vi "MicosCore.vi"(5 "NumOfAxis":i32=3, 6 "MotorDisabled":refnum<vi>, 7 "Simulation":bool, 8 "error in":errorcluster, 9 "Serial Configuration":T1={"Baud Rate"=115200, "Parity"=0, "Data Bits"=8, "Stop Bits"=10, "Flow Control"=0} {"Flow Control" items=["None", "XON/XOFF", "RTS/CTS", "XON/XOFF & RTS/CTS", "DTR/DSR", "XON/XOFF & DTR/DSR"]; "Stop Bits" items=["1.0"=10, "1.5"=15, "2.0"=20]; "Data Bits" items=["7"=7, "8"=8]; "Parity" items=["None", "Odd", "Even", "Mark", "Space"]; "Baud Rate" items=["300"=300, "600"=600, "1200"=1200, "2400"=2400, "4800"=4800, "9600"=9600, "19200"=19200]}, 10 "CommPort":refnum<visa-resource-name>, 11 "ControlQueue in":refnum<queue>) -> (0 "error out":errorcluster, 3 "queue out":refnum<queue>)   [LabVIEW 2012, in "Micos_uic.lvlib"]
uses:
  Micos_uic.lvlib
  Public/Data/Micos_State.ctl
  Public/Data/Micos_Data.ctl
  <vilib>/Utility/error.llb/DialogType.ctl
  Public/Position_Micos.vi
  user.lib/Utility/ErrorLog_lib.lvlib
panel:
  out "Numeric":i32
  out "appended array":u32[](array[numeric])
  in  "Go_MoveRel":bool caption="Go"
  out "WaitStopBlink":i32
  out "tick_start":u32
  out "tick_stop":u32
  out "Returned_String":string
  out "refresh rate":i32
  out "resfresh counter":i32
  in  "MotorDisabled":bool caption="Go"
  in  "Home":bool caption="Go"
  in  "StepWidth":dbl(ring)=0.2 items=["0.2 um"=0.0002, "0.001 mm"=0.001, "0.002 mm"=0.002, "0.005 mm "=0.005, "0.01 mm"=0.01, "0.02 mm"=0.02, "0.05 mm"=0.05, "0.1 mm"=0.1, "0.2 mm"=0.2, "1 mm"=1.0]
  in  "Z-":bool
  in  "Z+":bool
  in  "X+":bool
  in  "X-":bool
  in  "Y-":bool
  in  "Y+":bool
  in  "ClearErr":bool caption="Go"
  in  "STOP":bool caption="Go"
  in  "Quit":bool caption="Go"
  out "Instrument Driver Revision":string
  out "Instrument Firmware Revision":string
  in  "SetPosition":dbl[](array[numeric])=[1.0, 1.0, 1.0] caption="Position" format="%.4f"
  in  "SetVelocity":dbl[](array[numeric])=[1.0] caption="Velocity"
  in  "SetAcceleration":dbl[](array[numeric])=[50.0] caption="Acceleration"
  in  "Go":bool
  out "Moving":bool
  out "Acceleration":dbl[](array[numeric])
  out "Velocity":dbl[](array[numeric])
  out "Position":dbl[](array[numeric])
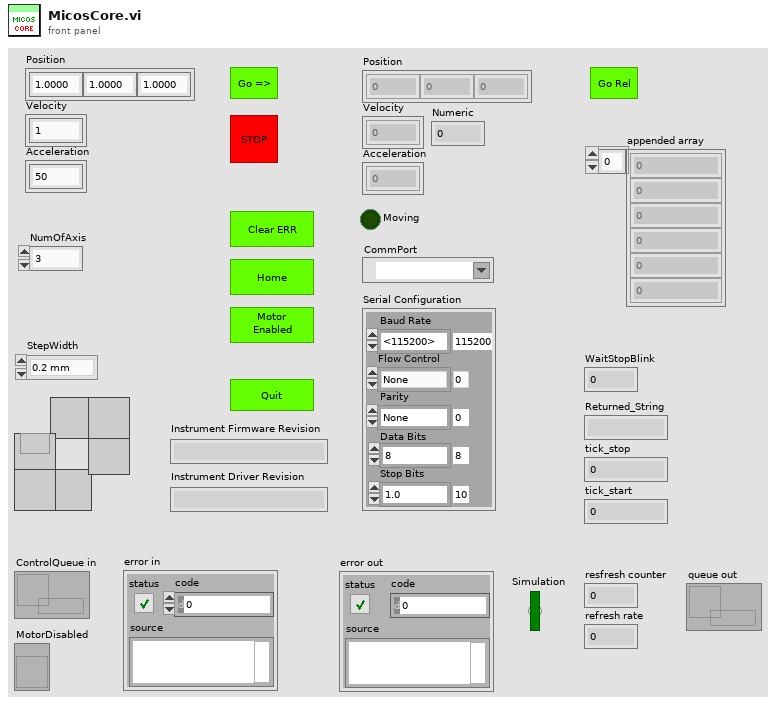
[diagram p1: front panel]
types:
  T1 = cluster{"Baud Rate":u32, "Parity":u16, "Data Bits":u16, "Stop Bits":u16, "Flow Control":u16}
  T2 = cluster{"CommPort":refnum<vi>, "Serial Configuration":refnum<vi>, "SetPosition":refnum<vi>, "SetAcceleration":refnum<vi>, "SetVelocity":refnum<vi>, "StepWidth":refnum<vi>, "WaitStopReturn_Queue":refnum<queue>}
  T3 = typedef "Micos_uic.lvlib/Micos_State.ctl" = cluster{"State":enum16{"Initialize", "SetDefaultConfig", "Close", "Quit", "Identify", "MoveAbs", "MoveAbs_all", "MoveRel", "MoveRel_all", "STOP", "Origin/Home", "WaitStop", "QueryStatus", "UpdateXPos", "UpdateAll", "SetVelocity", "SetAcceleration", "ClearErr", "LogMessage", "MotorEnable(1)", "EnableAxis", "JoyStick", "GetVelocity", "GetAcceleration", "SendCmd", "SetSoftLimits", "Beep", "_SettingReturn"}, "Params.":variant}
  T4 = typedef "Micos_uic.lvlib/Micos_Data.ctl" = cluster{"Position":dbl[], "Velocity":dbl[], "Acceleration":dbl[], "Moving":bool, "Simulation":bool, "tickcount_mov":u32, "tickcount_pos":u32, "NumOfAxis":i32, "Initialized":bool, "CommPort":refnum<visa-resource-name>, "Range":dbl[][], "Serial Configuration":cluster{"Baud Rate":u32, "Parity":u16, "Data Bits":u16, "Stop Bits":u16, "Flow Control":u16}, "MotorDisabled":refnum<vi>}
  T5 = enum16{"Initialize", "SetDefaultConfig", "Close", "Quit", "Identify", "MoveAbs", "MoveAbs_all", "MoveRel", "MoveRel_all", "STOP", "Origin/Home", "WaitStop", "QueryStatus", "UpdateXPos", "UpdateAll", "SetVelocity", "SetAcceleration", "ClearErr", "LogMessage", "MotorEnable(1)", "EnableAxis", "JoyStick", "GetVelocity", "GetAcceleration", "SendCmd", "SetSoftLimits", "Beep", "_SettingReturn"}
  T6 = cluster{"Acceleration":dbl[], "Velocity":dbl[], "tick_move_target":u32, "Position target":dbl[], "Velocity_axial":dbl[]}
  T7 = cluster{"Position_Target":dbl[], "Velocity_axial":dbl[], "Acceleration":dbl[], "Moving":bool, "Simulation":bool, "tick_MoveTarget":u32, "NumOfAxis":i32, "Range":dbl[][]}
  T8 = enum16{"Initialize", "SetDefaultConfig", "Close", "Quit", "Identify", "MoveAbs", "MoveAbs_all", "MoveRel", "MoveRel_all", "STOP", "Origin/Home", "WaitStop", "QueryStatus", "UpdateXPos", "UpdateAll", "SetVelocity", "SetAcceleration", "ClearErr", "LogMessage", "MotorEnable(1)", "EnableAxis", "JoyStick", "GetVelocity", "GetAcceleration", "SendCmd", "SetSoftLimits", "Beep", "_SettingReturn"}[]
  T9 = typedef "DialogType.ctl" = u16
  T10 = typedef "StepWidthSelector.ctl" = dbl
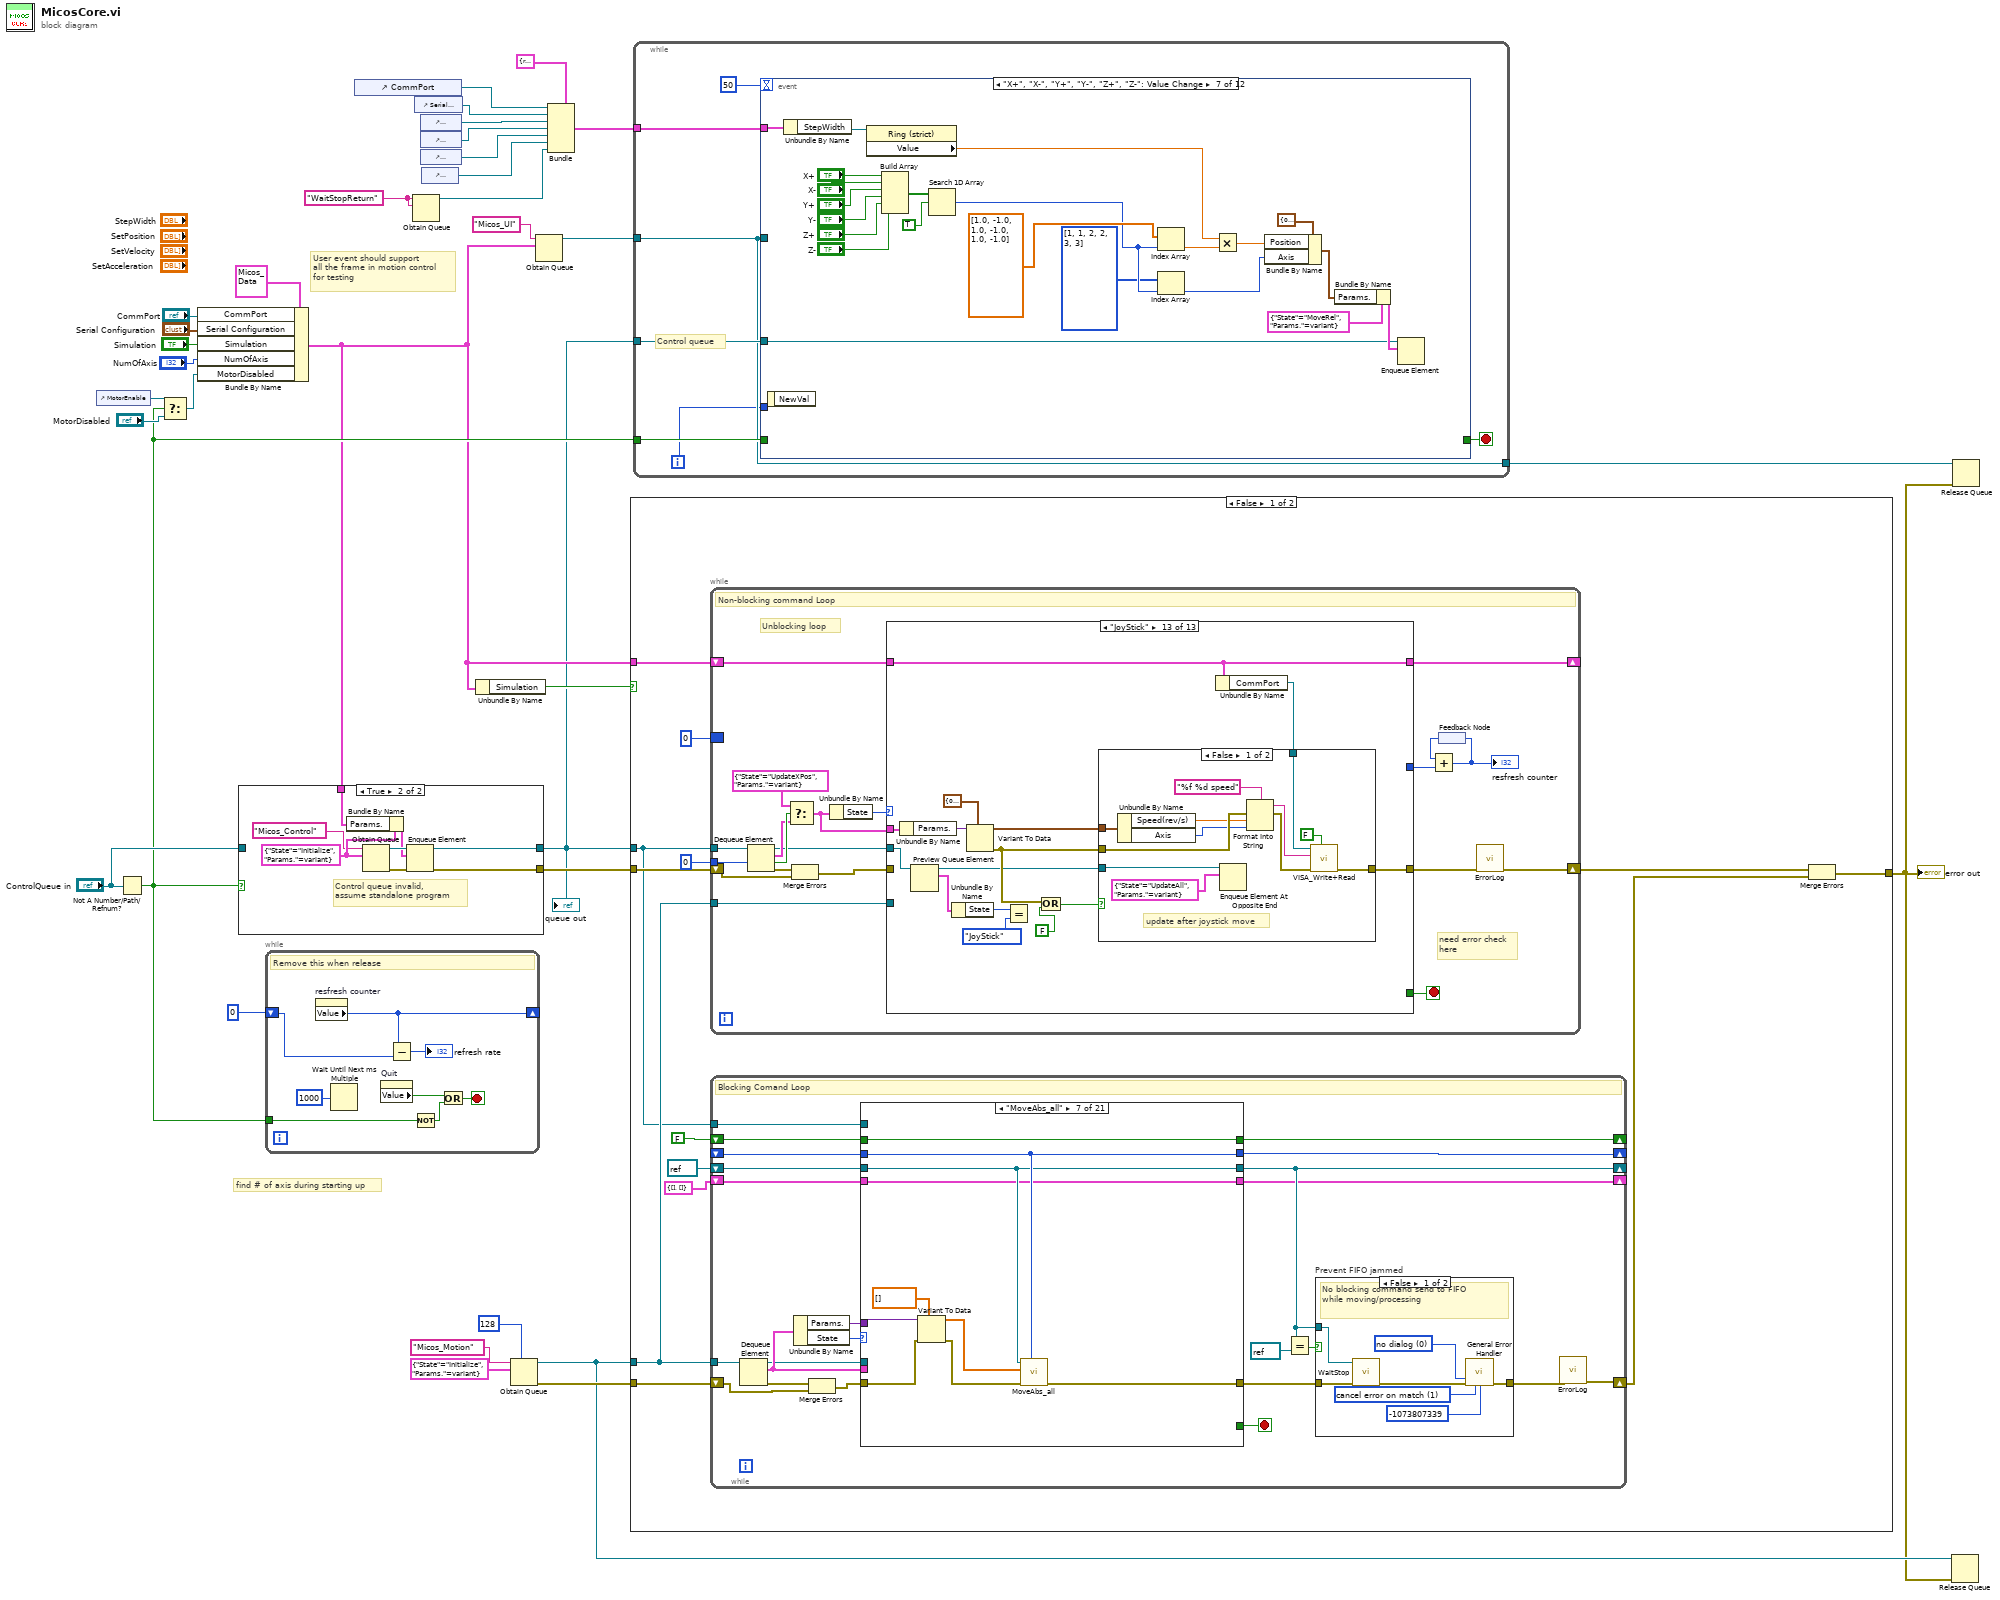
[diagram p0: block diagram]
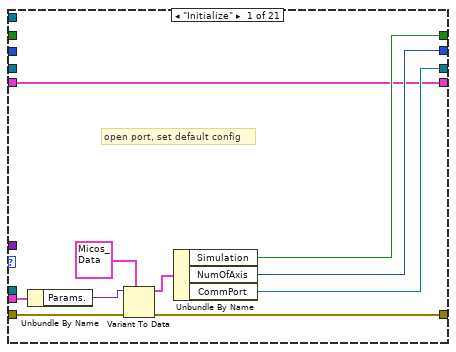
[diagram p3: hidden frame]
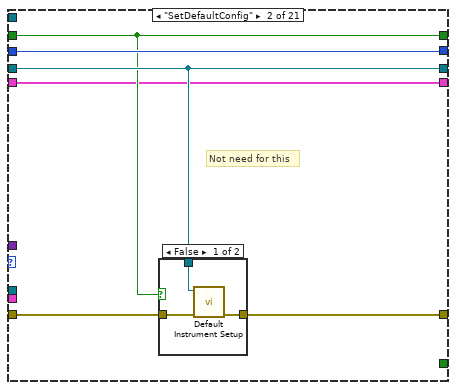
[diagram p4: hidden frame]
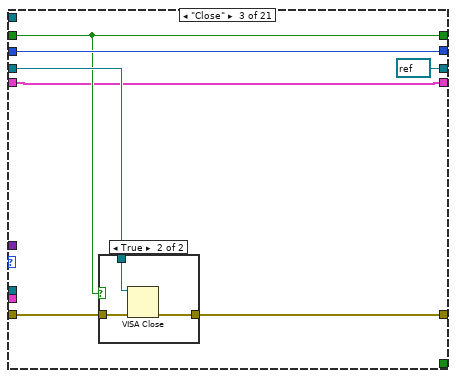
[diagram p6: hidden frame]
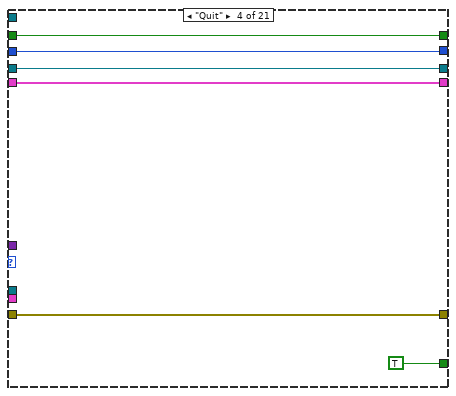
[diagram p8: hidden frame]
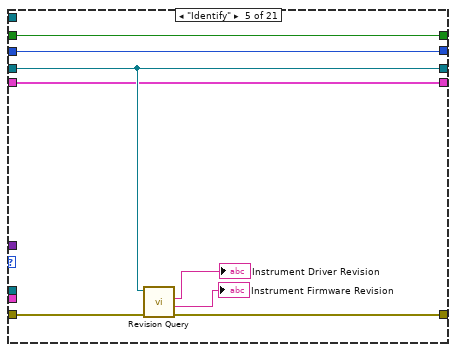
[diagram p9: hidden frame]
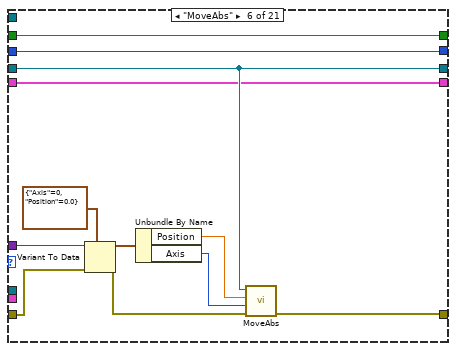
[diagram p10: hidden frame]
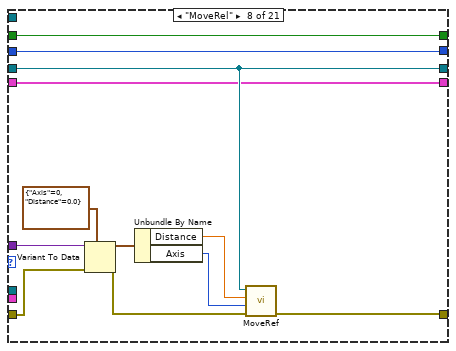
[diagram p11: hidden frame]
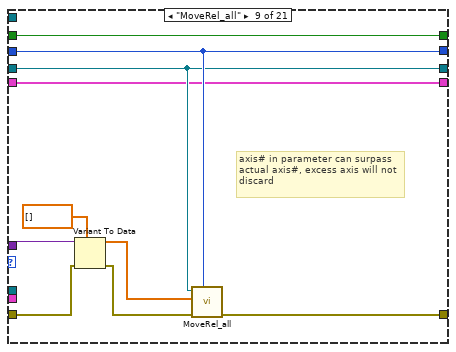
[diagram p12: hidden frame]
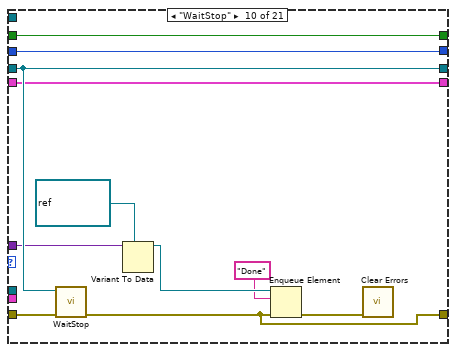
[diagram p13: hidden frame]
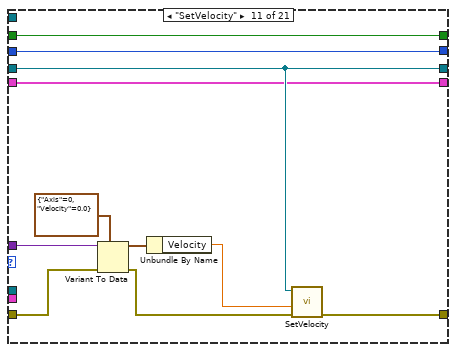
[diagram p14: hidden frame]
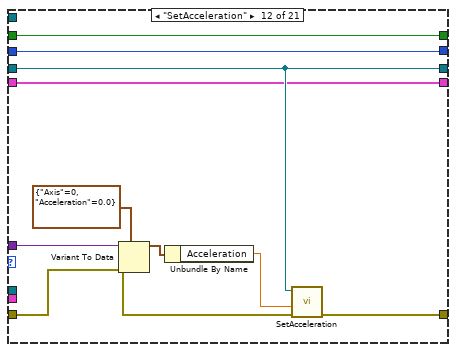
[diagram p15: hidden frame]
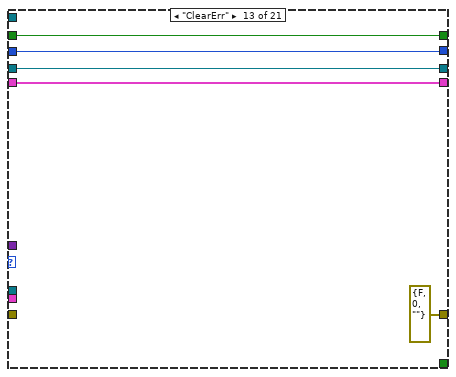
[diagram p16: hidden frame]
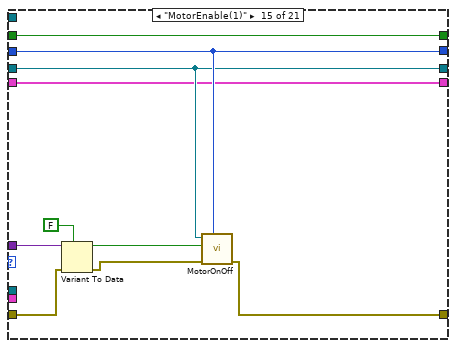
[diagram p18: hidden frame]
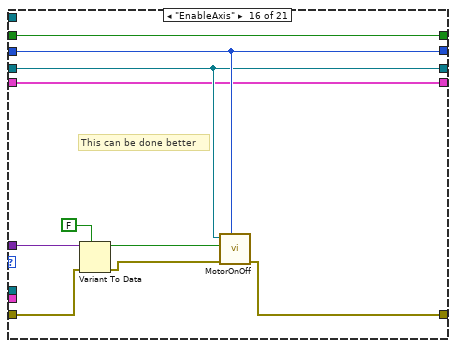
[diagram p19: hidden frame]
diagram:
  w8 = "WaitStopReturn" ("name (unnamed)")
  # "find # of axis during starting up"
  # "User event should support \nall the frame in motion control\nfor testing"
  n1 = control-ref of="MotorEnable"() -> (w16:refnum<vi>)
  n2 = Not A Number/Path/Refnum?(number/path/refnum="ControlQueue in") -> (NaN/Path/Refnum?=w11:bool)
  n3 = Select(t=w16, s=w11, f="MotorDisabled") -> (s? t:f=w14:refnum<vi>)
  n4 = Bundle By Name(cluster=T4 {"Position"=[], "Velocity"=[], "Acceleration"=[], "Moving"=FALSE, "Simulation"=FALSE, "tickcount_mov"=0, "tickcount_pos"=0, "NumOfAxis"=0, "Initialized"=FALSE, "CommPort"="", "Range"=[], "Serial Configuration"={"Baud Rate"=0, "Parity"=0, "Data Bits"=0, "Stop Bits"=0, "Flow Control"=0}, "MotorDisabled"=refnum}, "CommPort"="CommPort", "Serial Configuration"="Serial Configuration", "Simulation"="Simulation", "NumOfAxis"="NumOfAxis", "MotorDisabled"=w14) -> (w9:T4)
  n5 = case shown="True" w11 {
    tunnel: [w36 w42] -> w4
    tunnel: ["error in" w41] -> w34
    tunnel: "ControlQueue in" -> [w36 _]
    tunnel: w9 -> [_ w38]
    frame False {
    }
    frame True {
      w43 = T3 {"State"=enum."Initialize", "Params."=variant}
      # "Control queue invalid, \nassume standalone program"
      n6 = Bundle By Name(cluster=w43, "Params."=w38) -> (w39:T3)
      n7 = Obtain Queue(name (unnamed)="Micos_Control", element data type=w43) -> (queue out=w44:refnum<queue>, error out=w40:errorcluster)  [unwired: 3 in, 1 out]
      n8 = Enqueue Element(queue=w44, element=w39, error in (no error)=w40) -> (queue out=w42:refnum<queue>, error out=w41:errorcluster)  [unwired: 1 in, 1 out]
    }
  }
  "queue out" <- w4
  n9 = while {
    shift-right: [w49] -> _
    shift-left: 0 ("resfresh counter") -> [w52]
    tunnel: w11 -> [w46]
    stop <- w47 stop-if-true
    # "Remove this when release"
    n10 = property on="resfresh counter" class="DigNum (strict)"() -> ("Value"=w49:i32)  [unwired: 2 in, 2 out]
    n11 = Wait Until Next ms Multiple(millisecond multiple=u32 1000) -> ()  [unwired: 1 out]
    n12 = property on="Quit" class="Bool (strict)"() -> ("Value"=w50:bool)  [unwired: 2 in, 2 out]
    n13 = Subtract(x=w49, y=w52) -> (x-y=→"refresh rate":i32)
    n14 = Not(x=w46) -> (.not. x?=w45:bool)
    n15 = Or(x=w50, y=w45) -> (x .or. y?=w47:bool)
  }
  n16 = control-ref of="CommPort"() -> (w26:refnum<vi>)
  n17 = Obtain Queue(name (unnamed)=w8, element data type=w8) -> (queue out=w7:refnum<queue>)  [unwired: 3 in, 2 out]
  n18 = control-ref of="Serial Configuration"() -> (w27:refnum<vi>)
  n19 = control-ref of="SetPosition"() -> (w25:refnum<vi>)
  n20 = control-ref of="SetAcceleration"() -> (w24:refnum<vi>)
  n21 = control-ref of="SetVelocity"() -> (w23:refnum<vi>)
  n22 = control-ref of="StepWidth"() -> (w17:refnum<vi>)
  n23 = Unbundle By Name(w9) -> ("Simulation"=w10:bool)
  n24 = Obtain Queue(max queue size (-1, unlimited)=128, name (unnamed)="Micos_Motion", element data type=T3 {"State"=enum."Initialize", "Params."=variant}) -> (queue out=w2:refnum<queue>, error out=w31:errorcluster)  [unwired: 2 in, 1 out]
  n25 = Obtain Queue(name (unnamed)="Micos_UI", element data type=w9) -> (queue out=w5:refnum<queue>)  [unwired: 3 in, 2 out]
  n26 = Bundle(cluster=T2 {"CommPort"=refnum, "Serial Configuration"=refnum, "SetPosition"=refnum, "SetAcceleration"=refnum, "SetVelocity"=refnum, "StepWidth"=refnum, "WaitStopReturn_Queue"=refnum}, "CommPort"=w26, "Serial Configuration"=w27, "SetPosition"=w25, "SetAcceleration"=w24, "SetVelocity"=w23, "StepWidth"=w17, "WaitStopReturn_Queue"=w7) -> (w22:T2)
  n27 = case shown="False" w10 {
    tunnel: w34 -> [w65 w585]
    tunnel: w31 -> [w64 w584]
    tunnel: w2 -> [w63 w583]
    tunnel: w9 -> [w60 w577]
    tunnel: w4 -> [w57 w579]
    tunnel: [w54 w574] -> w1
    frame False {
      n28 = while {
        tunnel: w57 -> [w303]
        shift-right: [w313] -> _
        shift-left: w60 -> [w312]
        tunnel: w63 -> [w310]
        shift-right: [w294] -> w56
        shift-left: w65 -> [w299]
        tunnel: 0 ("f") -> [w301]
        border: 0 -> [_]
        stop <- w311 stop-if-true
        # "Unblocking loop"
        # "need error check\nhere"
        # "Non-blocking command Loop"
        n29 = Dequeue Element(queue=w303, timeout in ms (-1)=w301) -> (queue out=w304:refnum<queue>, element=w306:T3, timed out?=w308:bool, error out=w309:errorcluster)  [unwired: 1 in]
        n30 = Select(t=T3 {"State"=enum."UpdateXPos", "Params."=variant} ("element"), s=w308, f=w306) -> (s? t:f=w305:T3)
        n31 = Merge Errors(w309, w299) -> (w300:errorcluster)
        n32 = Unbundle By Name(w305) -> ("State"=w302:T5)
        n33 = case shown="\"JoyStick\"" w302 {
          tunnel: w305 -> [w321 w353 _ _ w408 _ _ _ _ w512 w531 w543 w556]
          tunnel: [w330 w350 w370 w394 w404 w413 w434 w471 w508 w517 w534 w541 w558] -> w313
          tunnel: w312 -> [w324 w348 w370 w394 w404 w413 w432 w469 w508 w517 w534 w544 w558]
          tunnel: [w320 _ TRUE _ _ _ _ _ _ _ _ _ _] -> w311
          tunnel: w310 -> [w315 w354 w373 w393 _ _ _ w458 _ w516 w533 _ _]
          tunnel: [w323 w351 w375 w389 w406 w411 w425 w461 errorcluster {"status"=FALSE, "code"=0, "source"=""} ("error out") w509 w530 w535 w559] -> w295
          tunnel: w300 -> [w327 w352 w371 w392 w407 w414 w433 w470 _ w515 w532 w536 _]
          tunnel: w304 -> [_ w346 _ _ _ _ w424 _ _ w513 _ _ w551]
          tunnel: [_ _ _ _ _ _ 1 1 _ _ _ _ _] -> w298
          frame "Initialize" {
            # "cmd +(stage data)"
            # "stage data"
            n34 = Unbundle By Name(w321) -> ("Params."=w328:variant)
            n35 = Variant To Data(error in=w327, type=w324, Variant=w328) -> (data=w325:T4, error out=w326:errorcluster)
            n36 = Select(t=w324, s=w326, f=w325) -> (s? t:f=w314:T4)
            n37 = Unbundle By Name(w314) -> ("Serial Configuration"=w322:T1, "CommPort"=w318:refnum<visa-resource-name>)
            n38 = call <vilib>:"Clear Errors.vi"("error in (no error)"=w326) -> ("error out"=w316:errorcluster)  [unwired: 6 in]
            n39 = Equal?(x=w318, y=refnum<visa-resource-name> refnum ("CommPort")) -> (x = y?=w319:bool)
            n40 = Bundle By Name(cluster=w314, "Initialized"=TRUE) -> (w330:T4)
            n41 = case shown="False" w319 {
              tunnel: w316 -> [w340 w343]
              tunnel: [w339 errorcluster {"status"=FALSE, "code"=-5104, "source"="Device unspecifiied,\nSkip execution"} ("error out")] -> w323
              tunnel: w322 -> [w338 _]
              tunnel: w318 -> [w337 _]
              tunnel: [_ w341] -> w320
              tunnel: w315 -> [w332 w345]
              tunnel: w314 -> [w331 _]
              frame False {
                n42 = Bundle By Name(cluster=T3 {"State"=enum."Initialize", "Params."=variant}, "Params."=w331) -> (w334:T3)
                n43 = call "Initialize.vi"("Serial Configuration"=w338, "error in (no error)"=w340, "Reset (True)"=FALSE, "ID Query (True)"=FALSE, "VISA resource name"=w337) -> ("error out"=w339:errorcluster)  [unwired: 5 in, 1 out]
                n44 = Enqueue Element(queue=w332, element=w334) -> ()  [unwired: 2 in, 3 out]
              }
              frame True {
                w341 = TRUE
                n45 = Enqueue Element(queue=w345, element=T3 {"State"=enum."Quit", "Params."=variant}, error in (no error)=w343) -> ()  [unwired: 1 in, 3 out]
                n46 = property on="Quit" class="Bool (strict)"("Val(Sgnl)"=w341) -> ()  [unwired: 2 in, 2 out]
              }
            }
          }
          frame "Close" {
            n47 = Unbundle By Name(w348) -> ("Moving"=w347:bool)
            n48 = case shown="True" w347 {
              tunnel: w354 -> [w358 _]
              tunnel: w353 -> [w357 w359]
              tunnel: w352 -> [w356 w363]
              tunnel: [w355 w360] -> w351
              tunnel: w346 -> [_ w368]
              frame False {
                n49 = Enqueue Element "Imply \"Close\""(queue=w358, element=w357, error in (no error)=w356) -> (error out=w355:errorcluster)  [unwired: 1 in, 2 out]
              }
              frame True {
                n50 = Enqueue Element At Opposite End "Implied \"Close\""(queue=w368, element=w359, error in (no error)=w363) -> (queue out=w367:refnum<queue>, error out=w362:errorcluster)  [unwired: 1 in, 1 out]
                n51 = Enqueue Element At Opposite End(queue=w367, element=T3 {"State"=enum."UpdateAll", "Params."=variant}, error in (no error)=w362) -> (queue out=w366:refnum<queue>, error out=w361:errorcluster)  [unwired: 1 in, 1 out]
                n52 = Enqueue Element At Opposite End(queue=w366, element=T3 {"State"=enum."STOP", "Params."=variant}, error in (no error)=w361) -> (error out=w360:errorcluster)  [unwired: 1 in, 2 out]
              }
            }
            n53 = Bundle By Name(cluster=w348, "Initialized"=FALSE) -> (w350:T4)
          }
          frame "Quit" {
            n54 = Unbundle By Name(w370) -> ("Initialized"=w369:bool)
            n55 = case shown="True" w369 {
              tunnel: [w379 w383] -> w374
              tunnel: w373 -> [w379 w382]
              tunnel: [w378 w381] -> w372
              tunnel: w371 -> [w378 w380]
              frame False {
              }
              frame True {
                n56 = Enqueue Element(queue=w382, element=T3 {"State"=enum."Close", "Params."=variant}, error in (no error)=w380) -> (queue out=w383:refnum<queue>, error out=w381:errorcluster)  [unwired: 1 in, 1 out]
              }
            }
            n57 = Enqueue Element(queue=w374, element=T3 {"State"=enum."Quit", "Params."=variant}, error in (no error)=w372) -> (error out=w375:errorcluster)  [unwired: 1 in, 2 out]
          }
          frame "STOP" {
            w385 = T8 [enum."WaitStop", enum."UpdateAll", enum."Close", enum."Quit", enum."SetVelocity"] items=["Initialize", "SetDefaultConfig", "Close", "Quit", "Identify", "MoveAbs", "MoveAbs_all", "MoveRel", "MoveRel_all", "STOP", "Origin/Home", "WaitStop", "QueryStatus", "UpdateXPos", "UpdateAll", "SetVelocity", "SetAcceleration", "ClearErr", "LogMessage", "MotorEnable(1)", "EnableAxis", "JoyStick", "GetVelocity", "GetAcceleration", "SendCmd", "SetSoftLimits", "Beep", "_SettingReturn"]
            # "should not dump wait for stop!!"
            # "send stop to controller, update"
            n58 = Unbundle By Name(w394) -> ("CommPort"=w391:refnum<visa-resource-name>)
            n59 = Flush Queue(queue=w393, error in (no error)=w392) -> (queue out=w386:refnum<queue>, remaining elements=w387:T3[], error out=w390:errorcluster)
            n60 = VISA Write(VISA resource name=w391, write buffer="\u0003\r\n" ("Substring"), error in (no error)=w390) -> (error out=w389:errorcluster)  [unwired: 2 out]
            n61 = for {
              tunnel: w387 -> [w400] mode=indexing
              tunnel: w386 -> [w399]
              tunnel: w385 -> [w397]
              n62 = Unbundle By Name(w400) -> ("State"=w398:T5)
              n63 = Equal?(x=w398, y=w397) -> (x = y?=w395:bool[])
              n64 = Or Array Elements(Boolean array=w395) -> (logical OR=w396:bool)
              n65 = case shown="True" w396 {
                tunnel: w400 -> [_ w402]
                tunnel: w399 -> [_ w401]
                frame False {
                }
                frame True {
                  n66 = Enqueue Element At Opposite End(queue=w401, element=w402) -> ()  [unwired: 2 in, 3 out]
                }
              }
            }
          }
          frame "QueryStatus" {
            # "return the value to queue"
            n67 = Unbundle By Name(w408) -> ("Params."=w410:variant)
            n68 = Variant To Data(error in=w407, type=refnum<queue> refnum ("queue out"), Variant=w410) -> (data=w405:refnum<queue>, error out=w409:errorcluster)
            n69 = Enqueue Element(queue=w405, element=w404, error in (no error)=w409) -> (error out=w406:errorcluster)  [unwired: 1 in, 2 out]
          }
          frame "Origin/Home" {
            # "The stage won't work, if not calibrated/homed,\nSo calibration has to be in the non-blocking loop\n\nAlso, during calibration, communication stop, causing error"
            n70 = Unbundle By Name(w413) -> ("CommPort"=w412:refnum<visa-resource-name>)
            n71 = call "OriginSearch.vi"("error in"=w414, "VISA resource"=w412) -> ("error out"=w411:errorcluster)  [unwired: 9 in]
          }
          frame "UpdateXPos" {
            n72 = Unbundle By Name(w432) -> ("NumOfAxis"=w418:i32, "CommPort"=w420:refnum<visa-resource-name>)
            n73 = feedback #1(0) -> (w428:i32)
            n74 = Increment(x=w428) -> (x+1=w429:i32)
            n75 = Quotient & Remainder(x=w429, y=16) -> (x-y*floor(x/y)=w426:i32)  [unwired: 1 out]
            n76 = feedback-in #1(w426) -> ()
            n77 = Equal To 0?(x=w426) -> (x = 0?=w423:bool)
            n78 = call "Update_xPos.vi"("NumOfAxis"=w418, "error in (no error)"=w433, "VISA resource name"=w420) -> ("error out"=w416:errorcluster, "x_Moving"=w421:bool, "Position"=w419:dbl[], "tickcount_pos"=w431:u32)  [unwired: 5 in]
            n79 = Compound Arithmetic op=OR(invert w421, w423) -> (w422:bool)
            n80 = case shown="Error" w416 {
              selector: w416 -> [w435 w442]
              tunnel: [w439 w445] -> w434
              tunnel: w432 -> [w438 w445]
              tunnel: w431 -> [w437 _]
              tunnel: w419 -> [w436 _]
              tunnel: [w435 w441] -> w415
              frame No Error {
                n81 = Bundle By Name(cluster=w438, "tickcount_pos"=w437, "Position"=w436) -> (w439:T4)
              }
              frame Error {
                w440 = T9 0 items=["no dialog", "OK message", "continue or stop message", "OK message + warnings", "continue/stop + warnings"] ("type of dialog (OK msg:1)")
                w443 = 1 items=["no exception", "cancel error on match", "set error on match"] ("[exception action] (none:0)")
                n82 = for {
                  shift-right: [w449] -> w441
                  shift-left: w442 -> [w450]
                  tunnel: w443 -> [w448]
                  tunnel: i32[] [85, -1073807252, 1] -> [w447] mode=indexing
                  tunnel: w440 -> [w446]
                  n83 = call <vilib>:"General Error Handler.vi"("type of dialog (OK msg:1)"=w446, "error in (no error)"=w450, "[exception action] (none:0)"=w448, "[exception code]"=w447) -> ("error out"=w449:errorcluster)  [unwired: 7 in, 4 out]
                }
              }
            }
            n84 = case shown="True" w422 {
              tunnel: [w451 w455] -> w425
              tunnel: w424 -> [_ w454]
              tunnel: w415 -> [w451 w452]
              frame False {
              }
              frame True {
                n85 = Enqueue Element At Opposite End(queue=w454, element=T3 {"State"=enum."UpdateAll", "Params."=variant}, error in (no error)=w452) -> (error out=w455:errorcluster)  [unwired: 1 in, 2 out]
              }
            }
          }
          frame "UpdateAll" {
            n86 = Unbundle By Name(w469) -> ("MotorDisabled"=w460:refnum<vi>, "NumOfAxis"=w468:i32, "CommPort"=w467:refnum<visa-resource-name>)
            n87 = call "Update_all.vi"("# axis"=w468, "error in (no error)"=w470, "VISA resource name"=w467) -> ("error out"=w462:errorcluster, "Moving"=w463:bool, "Currrent postion"=w466:dbl[], "tickcount_pos"=w465:u32, "MotorDisabled"=w456:bool)  [unwired: 4 in]
            n88 = property class="Bool (strict)"(reference=w460, "Blinking"=w456, "Value"=w456) -> (error out=w459:errorcluster)  [unwired: 1 in, 1 out]
            n89 = case shown="Error" w462 {
              selector: w462 -> [_ w495]
              tunnel: [w486 w498] -> w471
              tunnel: w469 -> [w485 w498]
              tunnel: w466 -> [w484 _]
              tunnel: w465 -> [w483 _]
              tunnel: w463 -> [w481 _]
              tunnel: [_ w494] -> w461
              tunnel: w458 -> [w482 _]
              tunnel: T3[] [{"State"=enum."GetVelocity", "Params."=variant}, {"State"=enum."GetAcceleration", "Params."=variant}, {"State"=enum."_SettingReturn", "Params."=variant}] -> [w480 _]
              frame No Error {
                w472 = FALSE  # Bypass continuous update
                n90 = Tick Count (ms)() -> (millisecond timer value=w478:u32)
                n91 = feedback #2() -> (w474:u32)  [unwired: 1 in]
                n92 = Subtract(x=w478, y=w474) -> (x-y=w477:u32)
                n93 = Greater?(x=u32 1000, y=w477) -> (0:w479:bool)
                n94 = Compound Arithmetic op=OR(w472, w481, w479) -> (w473:bool)
                n95 = Bundle By Name(cluster=w485, "tickcount_pos"=w483, "Position"=w484, "Moving"=w481) -> (w486:T4)
                n96 = case shown="True" w473 {
                  tunnel: w482 -> [w489 _]
                  tunnel: w480 -> [w488 _]
                  tunnel: [w487 w492] -> w475
                  tunnel: w474 -> [_ w492]
                  frame False {
                    n97 = for {
                      tunnel: w489 -> [w491]
                      tunnel: w488 -> [w490] mode=indexing
                      n98 = Enqueue Element(queue=w491, element=w490) -> ()  [unwired: 2 in, 3 out]
                    }
                    n99 = Tick Count (ms)() -> (millisecond timer value=w487:u32)
                  }
                  frame True {
                  }
                }
                n100 = feedback-in #2(w475) -> ()
              }
              frame Error {
                w493 = T9 0 items=["no dialog", "OK message", "continue or stop message", "OK message + warnings", "continue/stop + warnings"] ("type of dialog (OK msg:1)")
                w497 = 1 items=["no exception", "cancel error on match", "set error on match"] ("[exception action] (none:0)")
                n101 = disable-structure shown="Disabled" {
                  frame Disabled {
                    n102 = Tick Count (ms)() -> (millisecond timer value=w499:u32)
                    n103 = feedback #3() -> (w501:u32[])  [unwired: 1 in]
                    n104 = Build Array (concatenate)(w499, w501) -> (w500:u32[])
                    "appended array" <- w500
                    n105 = feedback-in #3(w500) -> ()
                  }
                  frame Enabled {
                  }
                }
                n106 = for {
                  shift-right: [w505] -> w494
                  shift-left: w495 -> [w506]
                  tunnel: w497 -> [w504]
                  tunnel: i32[] [85, -1073807252, -1073807339, 1] -> [w503] mode=indexing
                  tunnel: w493 -> [w502]
                  n107 = call <vilib>:"General Error Handler.vi"("type of dialog (OK msg:1)"=w502, "error in (no error)"=w506, "[exception action] (none:0)"=w504, "[exception code]"=w503) -> ("error out"=w505:errorcluster)  [unwired: 7 in, 4 out]
                }
              }
            }
            n108 = call <vilib>:"Clear Errors.vi"("error in (no error)"=w459) -> ()  [unwired: 6 in, 1 out]
          }
          frame "ClearErr" {
          }
          frame Default {
            # "system does not response \nafter a command is received"
            # "timeout push command back then do update?\n\npreventing blocking"
            n109 = Enqueue Element(queue=w516, element=w512, timeout in ms (-1)=0, error in (no error)=w515) -> (timed out?=w510:bool, error out=w511:errorcluster)  [unwired: 1 out]
            n110 = case shown="True" w510 {
              tunnel: w513 -> [_ w526]
              tunnel: w512 -> [_ w525]
              tunnel: w511 -> [w518 w524]
              tunnel: [w518 w521] -> w509
              frame False {
              }
              frame True {
                w519 = 500  # Prevent core stuck, but cause loosing command
                n111 = Enqueue Element At Opposite End(queue=w526, element=w525, timeout in ms (-1)=w519, error in (no error)=w524) -> (queue out=w523:refnum<queue>, error out=w520:errorcluster)  [unwired: 1 out]
                n112 = Enqueue Element At Opposite End(queue=w523, element=T3 {"State"=enum."UpdateXPos", "Params."=variant}, timeout in ms (-1)=w519, error in (no error)=w520) -> (error out=w521:errorcluster)  [unwired: 2 out]
              }
            }
          }
          frame "GetVelocity", "GetAcceleration" {
            # "system does not response \nafter a command is received"
            # "timeout push command back then do update?\n\npreventing blocking"
            n113 = Enqueue Element(queue=w533, element=w531, error in (no error)=w532) -> (queue out=w528:refnum<queue>, error out=w527:errorcluster)  [unwired: 1 in, 1 out]
            n114 = Enqueue Element(queue=w528, element=T3 {"State"=enum."_SettingReturn", "Params."=variant}, error in (no error)=w527) -> (error out=w530:errorcluster)  [unwired: 1 in, 2 out]
          }
          frame "_SettingReturn" {
            n115 = Unbundle By Name(w543) -> ("Params."=w542:variant)
            n116 = Variant To Data(error in=w536, type=cluster{"Acceleration":dbl[], "Velocity":dbl[]} {"Acceleration"=[], "Velocity"=[]}, Variant=w542) -> (data=w539:cluster{"Acceleration":dbl[], "Velocity":dbl[]}, error out=w535:errorcluster)
            n117 = Unbundle By Name(w539) -> ("Velocity"=w538:dbl[], "Acceleration"=w537:dbl[])
            n118 = Bundle By Name(cluster=w544, "Velocity"=w538, "Acceleration"=w537) -> (w541:T4)
          }
          frame "JoyStick" {
            n119 = Unbundle By Name(w556) -> ("Params."=w555:variant)
            n120 = Preview Queue Element(queue=w551) -> (queue out=w546:refnum<queue>, element=w549:T3)  [unwired: 2 in, 2 out]
            n121 = Unbundle By Name(w549) -> ("State"=w548:T5)
            n122 = Variant To Data(type=cluster{"Axis":i32, "Speed(rev/s)":dbl} {"Axis"=0, "Speed(rev/s)"=0.0}, Variant=w555) -> (data=w553:cluster{"Axis":i32, "Speed(rev/s)":dbl}, error out=w550:errorcluster)  [unwired: 1 in]
            n123 = Equal?(x=w548, y=T5."JoyStick" ("State")) -> ()  [unwired: 1 out]
            n124 = Or(x=w550, y=FALSE ("status")) -> (x .or. y?=w552:bool)
            n125 = Unbundle By Name(w558) -> ("CommPort"=w557:refnum<visa-resource-name>)
            n126 = case shown="False" w552 {
              tunnel: [w571 w572] -> w559
              tunnel: w557 -> [w569 _]
              tunnel: w553 -> [w568 _]
              tunnel: w550 -> [w564 w572]
              tunnel: w546 -> [w563 _]
              frame False {
                # "update after joystick move"
                n127 = Unbundle By Name(w568) -> ("Speed(rev/s)"=w561:dbl, "Axis"=w560:i32)
                n128 = Enqueue Element At Opposite End(queue=w563, element=T3 {"State"=enum."UpdateAll", "Params."=variant}) -> ()  [unwired: 2 in, 3 out]
                n129 = Format Into String(format string="%f %d speed", error in=w564, w561, w560) -> (resulting string=w567:string, error out=w566:errorcluster)  [unwired: 1 in]
                n130 = call "VISA_Write+Read.vi"("Read?"=FALSE, "error in (no error)"=w566, "Write Buffer"=w567, "VISA resource name"=w569) -> ("error out"=w571:errorcluster)  [unwired: 5 in, 2 out]
              }
              frame True {
              }
            }
          }
        }
        n131 = feedback #4() -> (w296:i32)
        n132 = Add(x=w296, y=w298) -> (x+y=w297:i32)
        "resfresh counter" <- w297
        n133 = feedback-in #4(w297) -> ()
        n134 = call "ErrorLog.vi"("error in (no error)"=w295) -> ("error out"=w294:errorcluster)  [unwired: 10 in]
      }
      n135 = while {
        tunnel: w63 -> [w78]
        shift-right: [w70] -> w53
        shift-left: w64 -> [w73]
        shift-right: [w75] -> _
        shift-left: refnum<visa-resource-name> refnum ("CommPort") -> [w79]
        shift-right: [w85] -> _
        shift-left: _ -> [w84]
        shift-right: [w81] -> _
        shift-left: FALSE -> [w82]
        tunnel: w57 -> [w69]
        shift-right: [w68] -> _
        shift-left: cluster{"Acceleration":dbl[], "Velocity":dbl[]} {"Acceleration"=[], "Velocity"=[]} -> [w67]
        stop <- w88 stop-if-true
        # "Blocking Comand Loop"
        n136 = Dequeue Element(queue=w78) -> (queue out=w66:refnum<queue>, element=w80:T3, error out=w87:errorcluster)  [unwired: 2 in, 1 out]
        n137 = Unbundle By Name(w80) -> ("Params."=w83:variant, "State"=w86:T5)
        n138 = Merge Errors(w87, w73) -> (w77:errorcluster)
        n139 = case shown="\"MoveAbs_all\"" w86 {
          tunnel: w80 -> [w106 _ _ _ _ _ _ _ _ _ _ _ _ _ _ _ _ _ _ _ w289]
          tunnel: [_ _ _ TRUE _ _ _ _ _ _ _ _ _ _ _ _ _ _ _ _ _] -> w88
          tunnel: [w103 w110 w121 w132 w138 w151 w163 w173 w185 w187 w202 w213 errorcluster {"status"=FALSE, "code"=0, "source"=""} ("error out") w228 w237 w242 w253 w255 w268 w277 w292] -> w72
          tunnel: w77 -> [w104 w111 w122 w132 w139 w148 w156 w170 w178 w194 w204 w215 _ w228 w236 w243 w253 w263 w274 w276 w292]
          tunnel: [w99 w109 refnum<visa-resource-name> refnum ("CommPort") w131 w137 w150 w161 w172 w183 w193 w206 w217 w222 w227 w232 w240 w252 w262 w273 w284 w293] -> w75
          tunnel: w79 -> [_ w109 w123 w131 w137 w150 w161 w172 w183 w193 w206 w217 w222 w227 w232 w240 w252 w262 w273 w284 w293]
          tunnel: w66 -> [_ _ _ _ _ _ _ _ _ _ _ _ _ _ _ _ _ _ _ _ _]
          tunnel: [w100 w112 w119 w130 w141 w153 w162 w175 w184 w196 w207 w218 w221 w226 w233 w241 w251 w261 w272 w283 w291] -> w85
          tunnel: w84 -> [_ w112 w119 w130 w141 w153 w162 w175 w184 w196 w207 w218 w221 w226 w233 w241 w251 w261 w272 w283 w291]
          tunnel: w83 -> [_ _ _ _ _ w149 w159 w171 w181 w192 w205 w216 _ _ w234 w244 _ _ _ _ _]
          tunnel: w82 -> [_ w108 w118 w129 w140 w152 w160 w174 w182 w195 w201 w212 w220 w225 w238 w248 w250 w264 w275 w282 w290]
          tunnel: [w98 w108 w118 w129 w140 w152 w160 w174 w182 w195 w201 w212 w220 w225 w238 w248 w250 w264 w275 w282 w290] -> w81
          tunnel: w69 -> [_ _ _ _ _ _ _ _ _ _ _ _ _ _ _ _ _ _ _ w281 _]
          tunnel: [w97 w107 w117 w128 w134 w142 w154 w164 w176 w186 w197 w208 w219 w224 w229 w239 w249 w260 w271 w278 w285] -> w68
          tunnel: w67 -> [w97 w107 w117 w128 w134 w142 w154 w164 w176 w186 w197 w208 w219 w224 w229 w239 w249 w259 w266 w278 w285]
          frame "Initialize" {
            # "open port, set default config"
            n140 = Unbundle By Name(w106) -> ("Params."=w105:variant)
            n141 = Variant To Data(error in=w104, type=T4 {"Position"=[], "Velocity"=[], "Acceleration"=[], "Moving"=FALSE, "Simulation"=FALSE, "tickcount_mov"=0, "tickcount_pos"=0, "NumOfAxis"=0, "Initialized"=FALSE, "CommPort"="", "Range"=[], "Serial Configuration"={"Baud Rate"=0, "Parity"=0, "Data Bits"=0, "Stop Bits"=0, "Flow Control"=0}, "MotorDisabled"=refnum}, Variant=w105) -> (data=w101:T4, error out=w103:errorcluster)
            n142 = Unbundle By Name(w101) -> ("Simulation"=w98:bool, "NumOfAxis"=w100:i32, "CommPort"=w99:refnum<visa-resource-name>)
          }
          frame "SetDefaultConfig" {
            # "Not need for this"
            n143 = case shown="False" w108 {
              tunnel: w111 -> [w115 w116]
              tunnel: [w114 w116] -> w110
              tunnel: w109 -> [w113 _]
              frame False {
                n144 = call "Default Instrument Setup.vi"("error in (no error)"=w115, "VISA resource name"=w113) -> ("error out"=w114:errorcluster)  [unwired: 8 in, 1 out]
              }
              frame True {
              }
            }
          }
          frame "Close" {
            n145 = case shown="True" w118 {
              tunnel: w123 -> [_ w127]
              tunnel: w122 -> [w124 w126]
              tunnel: [w124 w125] -> w121
              frame False {
              }
              frame True {
                n146 = VISA Close(VISA resource name=w127, error in (no error)=w126) -> (error out=w125:errorcluster)
              }
            }
          }
          frame "Quit" {
          }
          frame "Identify" {
            n147 = call "Revision Query.vi"("error in (no error)"=w139, "VISA resource name"=w137) -> ("error out"=w138:errorcluster, "Instrument Firmware Revision"=→"Instrument Firmware Revision":string, "Instrument Driver Revision"=→"Instrument Driver Revision":string)  [unwired: 6 in, 1 out]
          }
          frame "MoveAbs" {
            n148 = Variant To Data(error in=w148, type=cluster{"Axis":i32, "Position":dbl} {"Axis"=0, "Position"=0.0}, Variant=w149) -> (data=w145:cluster{"Axis":i32, "Position":dbl}, error out=w147:errorcluster)
            n149 = Unbundle By Name(w145) -> ("Position"=w143:dbl, "Axis"=w144:i32)
            n150 = call "MoveAbs.vi"("error in"=w147, "Axis"=w144, "Position"=w143, "VISA resource"=w150) -> ("error out"=w151:errorcluster)  [unwired: 7 in]
          }
          frame "MoveAbs_all" {
            n151 = Variant To Data(error in=w156, type=dbl[] [] ("Position"), Variant=w159) -> (data=w158:dbl[], error out=w155:errorcluster)
            n152 = call "MoveAbs_all.vi"("# axis"=w162, "error in (no error)"=w155, "Position"=w158, "VISA resource name"=w161) -> ("error out"=w163:errorcluster)  [unwired: 7 in]
          }
          frame "MoveRel" {
            n153 = Variant To Data(error in=w170, type=cluster{"Axis":i32, "Distance":dbl} {"Axis"=0, "Distance"=0.0}, Variant=w171) -> (data=w167:cluster{"Axis":i32, "Distance":dbl}, error out=w169:errorcluster)
            n154 = Unbundle By Name(w167) -> ("Distance"=w165:dbl, "Axis"=w166:i32)
            n155 = call "MoveRef.vi"("error in"=w169, "Axis"=w166, "Position"=w165, "VISA resource"=w172) -> ("error out"=w173:errorcluster)  [unwired: 7 in]
          }
          frame "MoveRel_all" {
            # "axis# in parameter can surpass\nactual axis#, excess axis will not\ndiscard"
            n156 = Variant To Data(error in=w178, type=dbl[] [] ("Position"), Variant=w181) -> (data=w180:dbl[], error out=w177:errorcluster)
            n157 = call "MoveRel_all.vi"("# axis"=w184, "error in (no error)"=w177, "Position"=w180, "VISA resource name"=w183) -> ("error out"=w185:errorcluster)  [unwired: 7 in]
          }
          frame "WaitStop" {
            n158 = call "WaitStop.vi"("error in (no error)"=w194, "VISA resource name"=w193) -> ("error out"=w187:errorcluster)  [unwired: 8 in, 1 out]
            n159 = Variant To Data(type=refnum<queue> refnum ("Feedback"), Variant=w192) -> (data=w190:refnum<queue>)  [unwired: 1 in, 1 out]
            n160 = Enqueue Element(queue=w190, element="Done", error in (no error)=w187) -> (error out=w188:errorcluster)  [unwired: 1 in, 2 out]
            n161 = call <vilib>:"Clear Errors.vi"("error in (no error)"=w188) -> ()  [unwired: 6 in, 1 out]
          }
          frame "SetVelocity" {
            n162 = Variant To Data(error in=w204, type=cluster{"Axis":i32, "Velocity":dbl} {"Axis"=0, "Velocity"=0.0}, Variant=w205) -> (data=w199:cluster{"Axis":i32, "Velocity":dbl}, error out=w203:errorcluster)
            n163 = Unbundle By Name(w199) -> ("Velocity"=w198:dbl)
            n164 = call "SetVelocity.vi"("error in"=w203, "Velocity"=w198, "VISA resource"=w206) -> ("error out"=w202:errorcluster)  [unwired: 8 in]
          }
          frame "SetAcceleration" {
            n165 = Variant To Data(error in=w215, type=cluster{"Axis":i32, "Acceleration":dbl} {"Axis"=0, "Acceleration"=0.0}, Variant=w216) -> (data=w210:cluster{"Axis":i32, "Acceleration":dbl}, error out=w214:errorcluster)
            n166 = Unbundle By Name(w210) -> ("Acceleration"=w209:dbl)
            n167 = call "SetAcceleration.vi"("error in"=w214, "Acceleration"=w209, "VISA resource"=w217) -> ("error out"=w213:errorcluster)  [unwired: 8 in]
          }
          frame "ClearErr" {
          }
          frame "LogMessage" {
          }
          frame "MotorEnable(1)" {
            n168 = Variant To Data(error in=w236, type=FALSE ("On/Off"), Variant=w234) -> (data=w230:bool, error out=w235:errorcluster)
            n169 = call "MotorOnOff.vi"("#Axis"=w233, "error in"=w235, "Enabled"=w230, "VISA resource"=w232) -> ("error out"=w237:errorcluster)  [unwired: 7 in]
          }
          frame "EnableAxis" {
            # "This can be done better"
            n170 = Variant To Data(error in=w243, type=FALSE ("On/Off"), Variant=w244) -> (data=w245:bool, error out=w247:errorcluster)
            n171 = call "MotorOnOff.vi"("#Axis"=w241, "error in"=w247, "Enabled"=w245, "VISA resource"=w240) -> ("error out"=w242:errorcluster)  [unwired: 7 in]
          }
          frame "JoyStick" {
          }
          frame "GetVelocity" {
            n172 = Unbundle By Name(w259) -> ("Velocity"=w257:dbl[])
            n173 = call "GetVelocity.vi"("error in (no error)"=w263, "VISA resource name"=w262) -> ("error out"=w255:errorcluster, "Velocity"=w254:dbl)  [unwired: 8 in]
            n174 = Initialize Array(w254, w261) -> (w256:dbl[])
            n175 = Select(t=w257, s=w255, f=w256) -> (s? t:f=w258:dbl[])
            n176 = Bundle By Name(cluster=w259, "Velocity"=w258) -> (w260:cluster{"Acceleration":dbl[], "Velocity":dbl[]})
          }
          frame "GetAcceleration" {
            n177 = Unbundle By Name(w266) -> ("Acceleration"=w269:dbl[])
            n178 = call "GetAcceleration.vi"("error in (no error)"=w274, "VISA resource name"=w273) -> ("error out"=w268:errorcluster, "Acceleration"=w265:dbl)  [unwired: 8 in]
            n179 = Initialize Array(w265, w272) -> (w267:dbl[])
            n180 = Select(t=w269, s=w268, f=w267) -> (s? t:f=w270:dbl[])
            n181 = Bundle By Name(cluster=w266, "Acceleration"=w270) -> (w271:cluster{"Acceleration":dbl[], "Velocity":dbl[]})
          }
          frame "_SettingReturn" {
            n182 = Bundle By Name(cluster=T3 {"State"=enum."_SettingReturn", "Params."=variant} ("element"), "Params."=w278) -> (w279:T3)
            n183 = Enqueue Element(queue=w281, element=w279, error in (no error)=w276) -> (error out=w277:errorcluster)  [unwired: 1 in, 2 out]
          }
          frame Default {
            n184 = Unbundle By Name(w289) -> ("State"=w287:T5)
            n185 = Format Into String(format string="\nUnsupported command:%d,\nDefault frame", w287) -> (resulting string=w288:string)  [unwired: 2 in, 1 out]
            n186 = One Button Dialog(message=w288) -> ()  [unwired: 1 in, 1 out]
          }
        }
        n187 = Equal?(x=w75, y=refnum<visa-resource-name> refnum ("CommPort")) -> (x = y?=w76:bool)
        n188 = case "Prevent FIFO jammed" shown="False" w76 {
          tunnel: w72 -> [w95 w96]
          tunnel: [w93 w96] -> w71
          tunnel: w75 -> [w94 _]
          frame False {
            w89 = T9 0 items=["no dialog", "OK message", "continue or stop message", "OK message + warnings", "continue/stop + warnings"] ("type of dialog (OK msg:1)")
            w90 = 1 items=["no exception", "cancel error on match", "set error on match"] ("[exception action] (none:0)")
            # "No blocking command send to FIFO\nwhile moving/processing"
            n189 = call "WaitStop.vi"("error in (no error)"=w95, "VISA resource name"=w94) -> ("error out"=w92:errorcluster)  [unwired: 8 in, 1 out]
            n190 = call <vilib>:"General Error Handler.vi"("type of dialog (OK msg:1)"=w89, "error in (no error)"=w92, "[exception action] (none:0)"=w90, "[exception code]"=-1073807339) -> ("error out"=w93:errorcluster)  [unwired: 7 in, 4 out]
          }
          frame True {
          }
        }
        n191 = call "ErrorLog.vi"("error in (no error)"=w71) -> ("error out"=w70:errorcluster)  [unwired: 10 in]
      }
      n192 = Merge Errors(w56, w53) -> (w54:errorcluster)
    }
    frame True {
      n193 = while {
        tunnel: w579 -> [w890]
        shift-right: [w900] -> _
        shift-left: w577 -> [w899]
        tunnel: w583 -> [w897]
        shift-right: [w885] -> w578
        shift-left: w585 -> [w886]
        tunnel: 0 ("f") -> [w888]
        shift-right: [w884] -> _
        shift-left: T7 {"Position_Target"=[], "Velocity_axial"=[], "Acceleration"=[], "Moving"=FALSE, "Simulation"=FALSE, "tick_MoveTarget"=0, "NumOfAxis"=0, "Range"=[]} ("output cluster") -> [w883]
        stop <- w898 stop-if-true
        # "Unblocking loop"
        # "Non-blocking command Loop"
        n194 = Dequeue Element(queue=w890, timeout in ms (-1)=w888) -> (queue out=w891:refnum<queue>, element=w893:T3, timed out?=w895:bool, error out=w896:errorcluster)  [unwired: 1 in]
        n195 = Select(t=T3 {"State"=enum."UpdateXPos", "Params."=variant} ("element"), s=w895, f=w893) -> (s? t:f=w892:T3)
        n196 = Merge Errors(w896, w886) -> (w887:errorcluster)
        n197 = Unbundle By Name(w892) -> ("State"=w889:T5)
        n198 = case shown="Default" w889 {
          tunnel: w892 -> [w912 w927 _ _ w988 w1001 _ _ _ w1079 w1096 w1103]
          tunnel: [w903 w924 w945 w966 w993 w997 w1023 w1054 w1073 w1082 w1086 w1108] -> w900
          tunnel: w899 -> [w914 w922 w945 w964 w984 w997 w1021 w1052 w1073 w1082 w1097 w1108]
          tunnel: [_ _ TRUE _ _ _ _ _ _ _ _ _] -> w898
          tunnel: w897 -> [w911 w928 w948 w973 w985 _ _ _ _ w1081 _ w1107]
          tunnel: [w913 w925 w950 w971 w986 w999 w1015 w1053 errorcluster {"status"=FALSE, "code"=0, "source"=""} ("error out") w1078 w1090 w1100] -> w885
          tunnel: w887 -> [w917 w926 w946 w972 w987 w1000 w1022 w1053 _ w1080 w1091 w1106]
          tunnel: w891 -> [_ w920 _ _ _ _ w1014 _ _ _ _ w1104]
          tunnel: [w904 w919 w943 w967 w992 w995 w1010 w1050 w1071 w1074 w1089 w1099] -> w884
          tunnel: w883 -> [w910 w919 w943 w968 w994 w995 w1010 w1050 w1071 w1074 w1092 w1099]
          frame "Initialize" {
            # "cmd +(stage data)"
            # "stage data"
            n199 = Unbundle By Name(w912) -> ("Params."=w918:variant)
            n200 = Variant To Data(error in=w917, type=w914, Variant=w918) -> (data=w915:T4, error out=w916:errorcluster)
            n201 = Select(t=w914, s=w916, f=w915) -> (s? t:f=w906:T4)
            n202 = call <vilib>:"Clear Errors.vi"("error in (no error)"=w916) -> ("error out"=w913:errorcluster)  [unwired: 6 in]
            n203 = Unbundle By Name(w906) -> ("NumOfAxis"=w905:i32)
            n204 = Initialize Array(-1.2345 ("element"), w905) -> (w902:dbl[])
            n205 = global write "Position_Micos.vi" "Position_Micos"(w902) -> ()
            n206 = Bundle By Name(cluster=w910, "Position_Target"=w902) -> (w904:T7)
            n207 = Bundle By Name(cluster=w906, "Position"=w902, "Initialized"=TRUE) -> (w903:T4)
            n208 = Bundle By Name(cluster=T3 {"State"=enum."Initialize", "Params."=variant}, "Params."=w906) -> (w909:T3)
            n209 = Enqueue Element(queue=w911, element=w909) -> ()  [unwired: 2 in, 3 out]
          }
          frame "Close" {
            n210 = Unbundle By Name(w922) -> ("Moving"=w921:bool)
            n211 = case shown="True" w921 {
              tunnel: w928 -> [w932 _]
              tunnel: w927 -> [w931 w933]
              tunnel: w926 -> [w930 w937]
              tunnel: [w929 w934] -> w925
              tunnel: w920 -> [_ w942]
              frame False {
                n212 = Enqueue Element(queue=w932, element=w931, error in (no error)=w930) -> (error out=w929:errorcluster)  [unwired: 1 in, 2 out]
              }
              frame True {
                n213 = Enqueue Element At Opposite End(queue=w942, element=w933, error in (no error)=w937) -> (queue out=w941:refnum<queue>, error out=w936:errorcluster)  [unwired: 1 in, 1 out]
                n214 = Enqueue Element At Opposite End(queue=w941, element=T3 {"State"=enum."UpdateAll", "Params."=variant}, error in (no error)=w936) -> (queue out=w940:refnum<queue>, error out=w935:errorcluster)  [unwired: 1 in, 1 out]
                n215 = Enqueue Element At Opposite End(queue=w940, element=T3 {"State"=enum."STOP", "Params."=variant}, error in (no error)=w935) -> (error out=w934:errorcluster)  [unwired: 1 in, 2 out]
              }
            }
            n216 = Bundle By Name(cluster=w922, "Initialized"=FALSE) -> (w924:T4)
          }
          frame "Quit" {
            n217 = Unbundle By Name(w945) -> ("Initialized"=w944:bool)
            n218 = case shown="False" w944 {
              tunnel: [w954 w958] -> w949
              tunnel: w948 -> [w954 w957]
              tunnel: [w953 w956] -> w947
              tunnel: w946 -> [w953 w955]
              frame False {
              }
              frame True {
                n219 = Enqueue Element(queue=w957, element=T3 {"State"=enum."Close", "Params."=variant}, error in (no error)=w955) -> (queue out=w958:refnum<queue>, error out=w956:errorcluster)  [unwired: 1 in, 1 out]
              }
            }
            n220 = Enqueue Element(queue=w949, element=T3 {"State"=enum."Quit", "Params."=variant}, error in (no error)=w947) -> (error out=w950:errorcluster)  [unwired: 1 in, 2 out]
          }
          frame "STOP" {
            # "should not dump wait for stop!!"
            # "send stop to controller, update"
            n221 = Flush Queue(queue=w973, error in (no error)=w972) -> (queue out=w969:refnum<queue>, remaining elements=w970:T3[], error out=w971:errorcluster)
            n222 = for {
              tunnel: w970 -> [w979] mode=indexing
              shift-right: [w974] -> w961
              shift-left: w969 -> [w978]
              tunnel: [w974] -> _ mode=indexing
              n223 = Unbundle By Name(w979) -> ("State"=w977:T5)
              n224 = Equal?(x=w977, y=T5."WaitStop") -> (x = y?=w975:bool)
              n225 = case shown="True" w975 {
                tunnel: w979 -> [_ w983]
                tunnel: w978 -> [w980 w982]
                tunnel: [w980 w981] -> w974
                frame False {
                }
                frame True {
                  n226 = Enqueue Element At Opposite End(queue=w982, element=w983) -> (queue out=w981:refnum<queue>)  [unwired: 2 in, 2 out]
                }
              }
            }
            n227 = Unbundle By Name(w964) -> ("Position"=w963:dbl[])
            n228 = Tick Count (ms)() -> (millisecond timer value=w962:u32)
            n229 = Bundle By Name(cluster=w968, "tick_MoveTarget"=w962, "Position_Target"=w963) -> (w967:T7)
            n230 = Bundle By Name(cluster=w964, "Position"=w963, "Moving"=FALSE) -> (w966:T4)
            n231 = Enqueue Element At Opposite End "Has to be PUSH"(queue=w961, element=T3 {"State"=enum."STOP", "Params."=variant}) -> ()  [unwired: 2 in, 3 out]
          }
          frame "Origin/Home" {
            n232 = Enqueue Element(queue=w985, element=w988, error in (no error)=w987) -> (error out=w986:errorcluster)  [unwired: 1 in, 2 out]
            n233 = Unbundle By Name(w984) -> ("NumOfAxis"=w991:i32)
            n234 = Initialize Array(0.0 ("element"), w991) -> (w989:dbl[])
            n235 = Bundle By Name(cluster=w994, "Position_Target"=w989) -> (w992:T7)
            n236 = Bundle By Name(cluster=w984, "Position"=w989) -> (w993:T4)
          }
          frame "QueryStatus" {
            # "return the value to queue"
            n237 = Unbundle By Name(w1001) -> ("Params."=w1003:variant)
            n238 = Variant To Data(error in=w1000, type=refnum<queue> refnum ("queue out"), Variant=w1003) -> (data=w998:refnum<queue>, error out=w1002:errorcluster)
            n239 = Enqueue Element(queue=w998, element=w997, error in (no error)=w1002) -> (error out=w999:errorcluster)  [unwired: 1 in, 2 out]
          }
          frame "UpdateXPos" {
            # "target position - (target tickcount - current tickcount)*velocity = current position"
            n240 = Unbundle By Name(w1010) -> ("Position_Target"=w1009:dbl[], "tick_MoveTarget"=w1005:u32, "Velocity_axial"=w1011:dbl[])
            n241 = feedback #5(0) -> (w1018:i32)
            n242 = Increment(x=w1018) -> (x+1=w1019:i32)
            n243 = Quotient & Remainder(x=w1019, y=16) -> (x-y*floor(x/y)=w1016:i32)  [unwired: 1 out]
            n244 = feedback-in #5(w1016) -> ()
            n245 = Wait (ms) "Typical latency of Micos Corvus PCI"(milliseconds to wait=u32 6) -> ()  [unwired: 1 out]
            n246 = Equal To 0?(x=w1016) -> (x = 0?=w1013:bool)
            n247 = Tick Count (ms)() -> (millisecond timer value=w1006:u32)
            n248 = Less?(x=w1006, y=w1005) -> (x < y?=w1007:bool)
            n249 = case shown="True" w1007 {
              tunnel: [w1028 w1039] -> w1023
              tunnel: w1021 -> [w1027 w1038]
              tunnel: w1005 -> [_ w1037]
              tunnel: w1011 -> [_ w1035]
              tunnel: w1009 -> [w1025 w1032]
              tunnel: w1006 -> [w1026 w1031]
              tunnel: [w1024 w1029] -> w1004
              frame False {
                w1024 = FALSE ("Moving")
                # "Stopped"
                n250 = global write "Position_Micos.vi" "Moving"(w1024) -> ()
                n251 = global write "Position_Micos.vi" "Position_Micos"(w1025) -> ()
                n252 = Bundle By Name(cluster=w1027, "tickcount_pos"=w1026, "Position"=w1025, "Moving"=w1024) -> (w1028:T4)
              }
              frame True {
                w1029 = TRUE ("Moving")
                # "Moving"
                n253 = Subtract(x=w1037, y=w1031) -> (x-y=w1036:u32)
                n254 = Compound Arithmetic op=MULTIPLY(w1036, w1035, 0.001) -> (w1033:dbl[])
                n255 = Subtract(x=w1032, y=w1033) -> (x-y=w1030:dbl[])
                n256 = global write "Position_Micos.vi" "Moving"(w1029) -> ()
                n257 = Bundle By Name(cluster=w1038, "tickcount_pos"=w1031, "Position"=w1030, "Moving"=w1029) -> (w1039:T4)
                n258 = global write "Position_Micos.vi" "Position_Micos"(w1030) -> ()
              }
            }
            n259 = Compound Arithmetic op=OR(invert w1004, w1013) -> (w1012:bool)
            n260 = case shown="True" w1012 {
              tunnel: [w1040 w1044] -> w1015
              tunnel: w1014 -> [_ w1043]
              tunnel: w1022 -> [w1040 w1041]
              frame False {
              }
              frame True {
                n261 = Enqueue Element At Opposite End(queue=w1043, element=T3 {"State"=enum."UpdateAll", "Params."=variant}, error in (no error)=w1041) -> (error out=w1044:errorcluster)  [unwired: 1 in, 2 out]
              }
            }
          }
          frame "UpdateAll" {
            # "target position - (target tickcount - current tickcount)*velocity = current position"
            n262 = Unbundle By Name(w1050) -> ("Position_Target"=w1049:dbl[], "tick_MoveTarget"=w1045:u32, "Velocity_axial"=w1051:dbl[])
            n263 = Wait (ms) "Typical latency of Micos Corvus PCI"(milliseconds to wait=u32 6) -> ()  [unwired: 1 out]
            n264 = Tick Count (ms)() -> (millisecond timer value=w1046:u32)
            n265 = Greater Or Equal?(x=w1046, y=w1045) -> (x >= y?=w1047:bool)
            n266 = case shown="True" w1047 {
              tunnel: [w1065 w1070] -> w1054
              tunnel: w1052 -> [w1064 w1069]
              tunnel: w1045 -> [w1063 _]
              tunnel: w1051 -> [w1061 _]
              tunnel: w1049 -> [w1058 w1067]
              tunnel: w1046 -> [w1057 w1068]
              frame False {
                # "Generate current position"
                n267 = Subtract(x=w1063, y=w1057) -> (x-y=w1062:u32)
                n268 = Compound Arithmetic op=MULTIPLY(w1062, w1061, 0.001) -> (w1059:dbl[])
                n269 = Subtract(x=w1058, y=w1059) -> (x-y=w1056:dbl[])
                n270 = global write "Position_Micos.vi" "Position_Micos"(w1056) -> ()
                n271 = Bundle By Name(cluster=w1064, "tickcount_pos"=w1057, "Position"=w1056) -> (w1065:T4)
                n272 = global write "Position_Micos.vi" "Moving"(TRUE ("Moving")) -> ()
              }
              frame True {
                n273 = global write "Position_Micos.vi" "Position_Micos"(w1067) -> ()
                n274 = Bundle By Name(cluster=w1069, "tickcount_pos"=w1068, "Position"=w1067) -> (w1070:T4)
                n275 = global write "Position_Micos.vi" "Moving"(FALSE ("Moving")) -> ()
              }
            }
          }
          frame "ClearErr" {
          }
          frame "GetVelocity", "GetAcceleration" {
            # "system does not response \nafter a command is received"
            # "timeout push command back then do update?\n\npreventing blocking"
            n276 = Enqueue Element(queue=w1081, element=w1079, error in (no error)=w1080) -> (queue out=w1076:refnum<queue>, error out=w1075:errorcluster)  [unwired: 1 in, 1 out]
            n277 = Enqueue Element(queue=w1076, element=T3 {"State"=enum."_SettingReturn", "Params."=variant}, error in (no error)=w1075) -> (error out=w1078:errorcluster)  [unwired: 1 in, 2 out]
          }
          frame "_SettingReturn" {
            n278 = Unbundle By Name(w1096) -> ("Params."=w1095:variant)
            n279 = Variant To Data(error in=w1091, type=T6 {"Acceleration"=[], "Velocity"=[], "tick_move_target"=0, "Position target"=[], "Velocity_axial"=[]}, Variant=w1095) -> (data=w1093:T6, error out=w1090:errorcluster)
            n280 = Unbundle By Name(w1093) -> ("Position target"=w1088:dbl[], "Velocity_axial"=w1087:dbl[], "tick_move_target"=w1083:u32, "Velocity"=w1085:dbl[], "Acceleration"=w1084:dbl[])
            n281 = Bundle By Name(cluster=w1092, "Position_Target"=w1088, "Velocity_axial"=w1087, "tick_MoveTarget"=w1083) -> (w1089:T7)
            n282 = Bundle By Name(cluster=w1097, "Velocity"=w1085, "Acceleration"=w1084) -> (w1086:T4)
          }
          frame Default {
            # "system does not response \nafter a command is received"
            # "timeout push command back then do update?\n\npreventing blocking"
            n283 = Enqueue Element(queue=w1107, element=w1103, timeout in ms (-1)=50, error in (no error)=w1106) -> (timed out?=w1101:bool, error out=w1102:errorcluster)  [unwired: 1 out]
            n284 = case shown="True" w1101 {
              tunnel: w1104 -> [_ w1121]
              tunnel: w1103 -> [_ w1120]
              tunnel: w1102 -> [w1110 w1119]
              tunnel: [w1110 w1116] -> w1100
              tunnel: [_ w1111] -> w1098
              frame False {
              }
              frame True {
                w1114 = 50 ("timeout in ms (-1)")
                n285 = Enqueue Element At Opposite End(queue=w1121, element=w1120, timeout in ms (-1)=w1114, error in (no error)=w1119) -> (queue out=w1118:refnum<queue>, timed out?=w1112:bool, error out=w1115:errorcluster)
                n286 = Enqueue Element At Opposite End(queue=w1118, element=T3 {"State"=enum."UpdateXPos", "Params."=variant}, timeout in ms (-1)=w1114, error in (no error)=w1115) -> (timed out?=w1113:bool, error out=w1116:errorcluster)  [unwired: 1 out]
                n287 = Or(x=w1112, y=w1113) -> (x .or. y?=w1111:bool)
              }
            }
            n288 = case shown="True" w1098 {
              frame False {
              }
              frame True {
                n289 = One Button Dialog(message="queue full,time out,missing comand") -> ()  [unwired: 1 in, 1 out]
              }
            }
          }
        }
      }
      n290 = while {
        tunnel: w583 -> [w602]
        shift-right: [w599] -> w573
        shift-left: w584 -> [w600]
        shift-right: [w601] -> _
        shift-left: refnum<visa-resource-name> refnum ("CommPort") -> [w603]
        shift-right: [w609] -> _
        shift-left: _ -> [w608]
        shift-right: [w605] -> _
        shift-left: FALSE -> [w606]
        tunnel: w579 -> [w598]
        shift-right: [w597] -> _
        shift-left: T6 {"Acceleration"=[], "Velocity"=[], "tick_move_target"=0, "Position target"=[], "Velocity_axial"=[]} -> [w596]
        stop <- w611 stop-if-true
        w593 = T9 0 items=["no dialog", "OK message", "continue or stop message", "OK message + warnings", "continue/stop + warnings"] ("type of dialog (OK msg:1)")
        w594 = 1 items=["no exception", "cancel error on match", "set error on match"] ("[exception action] (none:0)")
        # "Blocking Comand Loop"
        n291 = Dequeue Element(queue=w602) -> (queue out=w586:refnum<queue>, element=w604:T3, error out=w610:errorcluster)  [unwired: 2 in, 1 out]
        n292 = Unbundle By Name(w604) -> ("Params."=w607:variant, "State"=w588:T5)
        n293 = Merge Errors(w610, w600) -> (w590:errorcluster)
        n294 = Not Equal?(x=T5."WaitStop", y=w588) -> (x != y?=w589:bool)
        n295 = case "Mimic Micos Behavior" shown="True" w589 {
          tunnel: w590 -> [w612 w615]
          tunnel: [w612 w614] -> w591
          tunnel: w586 -> [_ w613]
          frame False {
          }
          frame True {
            n296 = Enqueue Element At Opposite End(queue=w613, element=T3 {"State"=enum."WaitStop", "Params."=variant}, error in (no error)=w615) -> (error out=w614:errorcluster)  [unwired: 1 in, 2 out]
          }
        }
        n297 = case "Exeacuting commands" shown="\"WaitStop\"" w588 {
          tunnel: w604 -> [w635 _ _ _ _ _ _ _ _ _ _ _ _ _ _ _ _ _ _ _ _ _ w878]
          tunnel: [_ _ _ TRUE _ _ _ _ _ _ _ _ _ _ _ _ _ _ _ _ _ _ _] -> w611
          tunnel: [w620 w639 w645 w650 w654 w665 w686 w707 w734 w753 w763 w800 w812 errorcluster {"status"=FALSE, "code"=0, "source"=""} ("error out") w825 w831 w840 w846 w850 w855 w858 w873 w881] -> w592
          tunnel: w591 -> [w633 w639 w645 w650 w654 w671 w691 w717 w744 w754 w764 w801 w813 _ w825 w832 w837 w846 w850 w855 w857 w873 w881]
          tunnel: [w630 w638 refnum<visa-resource-name> refnum ("CommPort") w649 w653 w673 w693 w721 w748 w760 w774 w803 w815 w819 w824 w828 w835 w845 w849 w854 w865 w872 w882] -> w601
          tunnel: w603 -> [_ w638 _ w649 w653 w673 w693 w721 w748 w760 w774 w803 w815 w819 w824 w828 w835 w845 w849 w854 w865 w872 w882]
          tunnel: w586 -> [w623 _ _ _ _ w664 w685 w709 w736 w756 w762 _ _ _ _ _ _ _ _ _ _ _ _]
          tunnel: [w617 w640 w643 w648 w656 w668 w677 w722 w749 w759 w776 w792 w804 w818 w823 w829 w836 w844 w848 w853 w864 w867 w880] -> w609
          tunnel: w608 -> [_ w640 w643 w648 w656 w668 w677 w722 w749 w759 w776 w792 w804 w818 w823 w829 w836 w844 w848 w853 w864 w867 w880]
          tunnel: w607 -> [_ _ _ _ _ w672 w692 w719 w746 _ w773 w802 w814 _ _ w830 w838 _ _ _ _ _ _]
          tunnel: w606 -> [_ w637 w642 w647 w655 w674 w694 w720 w747 w758 w775 w799 w811 w817 w822 w833 w841 w843 w851 w856 w863 w871 w879]
          tunnel: [w629 w637 w642 w647 w655 w674 w694 w720 w747 w758 w775 w799 w811 w817 w822 w833 w841 w843 w851 w856 w863 w871 w879] -> w605
          tunnel: w598 -> [_ _ _ _ _ _ _ _ _ _ _ _ _ _ _ _ _ _ _ _ w862 _ _]
          tunnel: [w627 w636 w641 w646 w652 w669 w689 w715 w742 w752 w766 w796 w808 w816 w821 w826 w834 w842 w847 w852 w859 w869 w874] -> w597
          tunnel: w596 -> [w628 w636 w641 w646 w652 w669 w689 w716 w743 w757 w768 w797 w809 w816 w821 w826 w834 w842 w847 w852 w859 w870 w874]
          frame "Initialize" {
            # "open port, set default config"
            n298 = Unbundle By Name(w635) -> ("Params."=w634:variant)
            n299 = Variant To Data(error in=w633, type=T4 {"Position"=[], "Velocity"=[], "Acceleration"=[], "Moving"=FALSE, "Simulation"=FALSE, "tickcount_mov"=0, "tickcount_pos"=0, "NumOfAxis"=0, "Initialized"=FALSE, "CommPort"="", "Range"=[], "Serial Configuration"={"Baud Rate"=0, "Parity"=0, "Data Bits"=0, "Stop Bits"=0, "Flow Control"=0}, "MotorDisabled"=refnum}, Variant=w634) -> (data=w631:T4, error out=w621:errorcluster)
            n300 = Unbundle By Name(w631) -> ("Simulation"=w629:bool, "NumOfAxis"=w617:i32, "CommPort"=w630:refnum<visa-resource-name>)
            n301 = Enqueue Element At Opposite End(queue=w623, element=T3 {"State"=enum."_SettingReturn", "Params."=variant}, error in (no error)=w621) -> (error out=w620:errorcluster)  [unwired: 1 in, 2 out]
            n302 = Tick Count (ms)() -> (millisecond timer value=w624:u32)
            n303 = Initialize Array(-1.2345 ("element"), w617) -> (w618:dbl[])
            n304 = Initialize Array(1.0 ("element"), w617) -> (w625:dbl[])
            n305 = Bundle By Name(cluster=w628, "Position target"=w618, "Acceleration"=w625, "Velocity"=w625, "tick_move_target"=w624) -> (w627:T6)
          }
          frame "SetDefaultConfig" {
          }
          frame "Close" {
          }
          frame "Quit" {
          }
          frame "Identify" {
          }
          frame "MoveAbs" {
            n306 = Variant To Data(error in=w671, type=cluster{"Axis":i32, "Position":dbl} {"Axis"=0, "Position"=0.0}, Variant=w672) -> (data=w662:cluster{"Axis":i32, "Position":dbl}, error out=w666:errorcluster)
            n307 = global read "Position_Micos.vi" "Position_Micos"() -> (w661:dbl[])
            n308 = Unbundle By Name(w662) -> ("Axis"=w660:i32, "Position"=w658:dbl)
            n309 = Decrement(x=w660) -> (x-1=w659:i32)
            n310 = in-place {
              in-place-border: w658 -> [w675]
              n311 = in-place-array #6(w661, w659) -> ()  [unwired: 1 out]
              n312 = in-place-array #6(w675) -> (w657:dbl[])  [unwired: 1 out]
            }
            n313 = Bundle By Name(cluster=T3 {"State"=enum."MoveAbs_all", "Params."=variant} ("element"), "Params."=w657) -> (w663:T3)
            n314 = Enqueue Element At Opposite End(queue=w664, element=w663, error in (no error)=w666) -> (error out=w665:errorcluster)  [unwired: 1 in, 2 out]
          }
          frame "MoveRel" {
            n315 = Variant To Data(error in=w691, type=cluster{"Axis":i32, "Position":dbl} {"Axis"=0, "Position"=0.0}, Variant=w692) -> (data=w683:cluster{"Axis":i32, "Position":dbl}, error out=w687:errorcluster)
            n316 = Unbundle By Name(w683) -> ("Axis"=w682:i32, "Position"=w680:dbl)
            n317 = Initialize Array(0.0 ("element"), w677) -> (w676:dbl[])
            n318 = Decrement(x=w682) -> (x-1=w681:i32)
            n319 = in-place {
              in-place-border: w680 -> [w695]
              n320 = in-place-array #7(w676, w681) -> ()  [unwired: 1 out]
              n321 = in-place-array #7(w695) -> (w679:dbl[])  [unwired: 1 out]
            }
            n322 = Bundle By Name(cluster=T3 {"State"=enum."MoveRel_all", "Params."=variant} ("element"), "Params."=w679) -> (w684:T3)
            n323 = Enqueue Element At Opposite End(queue=w685, element=w684, error in (no error)=w687) -> (error out=w686:errorcluster)  [unwired: 1 in, 2 out]
          }
          frame "MoveRel_all" {
            n324 = global read "Position_Micos.vi" "Position_Micos"() -> (w696:dbl[])
            n325 = Variant To Data(error in=w717, type=dbl[] [] ("Position"), Variant=w719) -> (data=w698:dbl[], error out=w708:errorcluster)
            n326 = Add(x=w696, y=w698) -> (x+y=w697:dbl[])
            n327 = Absolute Value(x=w698) -> (abs(x)=w700:dbl[])
            n328 = Array Max & Min(array=w700) -> (max value=w699:dbl)  [unwired: 3 out]
            n329 = Unbundle By Name(w716) -> ("Velocity"=w703:dbl[])
            n330 = Index Array(array=w703) -> (element=w702:dbl)  [unwired: 1 in]
            n331 = Reciprocal(x=w699) -> (1/x=w713:dbl)
            n332 = Reciprocal(x=w702) -> (1/x=w701:dbl)
            n333 = Tick Count (ms)() -> (millisecond timer value=w710:u32)
            n334 = Enqueue Element At Opposite End(queue=w709, element=T3 {"State"=enum."_SettingReturn", "Params."=variant}, error in (no error)=w708) -> (error out=w707:errorcluster)  [unwired: 1 in, 2 out]
            n335 = Compound Arithmetic op=MULTIPLY(w701, w699, 1000.0 ("value")) -> (w711:dbl)
            n336 = To Unsigned Long Integer(number=w711) -> (unsigned 32bit integer=w705:u32)
            n337 = Compound Arithmetic op=MULTIPLY(w703, w698, w713) -> (w714:dbl[])
            n338 = Add(x=w710, y=w705) -> (x+y=w712:u32)
            n339 = Bundle By Name(cluster=w716, "Position target"=w697, "Velocity_axial"=w714, "tick_move_target"=w712) -> (w715:T6)
          }
          frame "MoveAbs_all" {
            n340 = global read "Position_Micos.vi" "Position_Micos"() -> (w725:dbl[])
            n341 = Variant To Data(error in=w744, type=dbl[] [] ("Position"), Variant=w746) -> (data=w724:dbl[], error out=w735:errorcluster)
            n342 = Subtract(x=w724, y=w725) -> (x-y=w723:dbl[])
            n343 = Absolute Value(x=w723) -> (abs(x)=w727:dbl[])
            n344 = Unbundle By Name(w743) -> ("Velocity"=w730:dbl[])
            n345 = Array Max & Min(array=w727) -> (max value=w726:dbl)  [unwired: 3 out]
            n346 = Index Array(array=w730) -> (element=w729:dbl)  [unwired: 1 in]
            n347 = Reciprocal(x=w726) -> (1/x=w740:dbl)
            n348 = Reciprocal(x=w729) -> (1/x=w728:dbl)
            n349 = Enqueue Element At Opposite End(queue=w736, element=T3 {"State"=enum."_SettingReturn", "Params."=variant}, error in (no error)=w735) -> (error out=w734:errorcluster)  [unwired: 1 in, 2 out]
            n350 = Tick Count (ms)() -> (millisecond timer value=w737:u32)
            n351 = Compound Arithmetic op=MULTIPLY(w728, w726, 1000.0 ("value")) -> (w738:dbl)
            n352 = To Unsigned Long Integer(number=w738) -> (unsigned 32bit integer=w732:u32)
            n353 = Compound Arithmetic op=MULTIPLY(w730, w723, w740) -> (w741:dbl[])
            n354 = Add(x=w737, y=w732) -> (x+y=w739:u32)
            n355 = Bundle By Name(cluster=w743, "Position target"=w724, "Velocity_axial"=w741, "tick_move_target"=w739) -> (w742:T6)
          }
          frame "STOP" {
            # "Simulation only"
            # "Only for simulation, \nFor dumping the stop command left in queue."
            n356 = Enqueue Element At Opposite End(queue=w756, element=T3 {"State"=enum."_SettingReturn", "Params."=variant}, error in (no error)=w754) -> (error out=w753:errorcluster)  [unwired: 1 in, 2 out]
            n357 = global read "Position_Micos.vi" "Position_Micos"() -> (w750:dbl[])
            n358 = Tick Count (ms)() -> (millisecond timer value=w751:u32)
            n359 = Bundle By Name(cluster=w757, "tick_move_target"=w751, "Position target"=w750) -> (w752:T6)
          }
          frame "WaitStop" {
            n360 = Unbundle By Name(w768) -> ("tick_move_target"=w767:u32)
            n361 = Variant To Data(error in=w764, type=refnum<queue> refnum ("Feedback"), Variant=w773) -> (data=w771:refnum<queue>, error out=w761:errorcluster)
            n362 = while {
              tunnel: w762 -> [w777]
              tunnel: w767 -> [w789]
              tunnel: [w782] -> w765
              i -> [w781]
              stop <- w785 stop-if-true
              n363 = Preview Queue Element(queue=w777, timeout in ms (-1)=0) -> (element=w788:T3, timed out?=w778:bool)  [unwired: 1 in, 2 out]
              n364 = Unbundle By Name(w788) -> ("State"=w787:T5)
              n365 = Tick Count (ms)() -> (millisecond timer value=w790:u32)
              n366 = Equal?(x=T5."STOP" ("State"), y=w787) -> (x = y?=w783:bool)
              n367 = Greater Or Equal?(x=w790, y=w789) -> (x >= y?=w784:bool)
              n368 = Compound Arithmetic op=AND(w783, invert w778) -> (w779:bool)
              n369 = Select(t=w790, s=w779, f=w789) -> (s? t:f=w782:u32)
              n370 = Wait Until Next ms Multiple(millisecond multiple=u32 50) -> ()  [unwired: 1 out]
              n371 = Or(x=w784, y=w779) -> (x .or. y?=w785:bool)
              "WaitStopBlink" <- w781
            }
            n372 = Bundle By Name(cluster=w768, "tick_move_target"=w765) -> (w766:T6)
            n373 = Enqueue Element(queue=w771, element="Done", error in (no error)=w761) -> (error out=w769:errorcluster)  [unwired: 1 in, 2 out]
            n374 = call <vilib>:"Clear Errors.vi"("error in (no error)"=w769) -> ("error out"=w763:errorcluster)  [unwired: 6 in]
          }
          frame "SetVelocity" {
            n375 = Variant To Data(error in=w801, type=cluster{"Axis":i32, "Velocity":dbl} {"Axis"=0, "Velocity"=0.0}, Variant=w802) -> (data=w795:cluster{"Axis":i32, "Velocity":dbl}, error out=w800:errorcluster)
            n376 = Unbundle By Name(w795) -> ("Velocity"=w793:dbl)
            n377 = Initialize Array(w793, w792) -> (w794:dbl[])
            n378 = Bundle By Name(cluster=w797, "Velocity"=w794) -> (w796:T6)
          }
          frame "SetAcceleration" {
            n379 = Variant To Data(error in=w813, type=cluster{"Axis":i32, "Acceleration":dbl} {"Axis"=0, "Acceleration"=0.0}, Variant=w814) -> (data=w807:cluster{"Axis":i32, "Acceleration":dbl}, error out=w812:errorcluster)
            n380 = Unbundle By Name(w807) -> ("Acceleration"=w805:dbl)
            n381 = Initialize Array(w805, w804) -> (w806:dbl[])
            n382 = Bundle By Name(cluster=w809, "Acceleration"=w806) -> (w808:T6)
          }
          frame "ClearErr" {
          }
          frame "LogMessage" {
          }
          frame "MotorEnable(1)" {
            n383 = Variant To Data(error in=w832, type=FALSE ("On/Off"), Variant=w830) -> (error out=w831:errorcluster)  [unwired: 1 out]
          }
          frame "EnableAxis" {
            n384 = Variant To Data(error in=w837, type=FALSE ("On/Off"), Variant=w838) -> (error out=w840:errorcluster)  [unwired: 1 out]
          }
          frame "JoyStick" {
          }
          frame "GetVelocity" {
            # "Send SettingReturn is taken cared in calling loop."
          }
          frame "GetAcceleration" {
            # "Send SettingReturn is taken cared in calling loop."
          }
          frame "_SettingReturn" {
            n385 = Bundle By Name(cluster=T3 {"State"=enum."_SettingReturn", "Params."=variant} ("element"), "Params."=w859) -> (w860:T3)
            n386 = Enqueue Element(queue=w862, element=w860, error in (no error)=w857) -> (error out=w858:errorcluster)  [unwired: 1 in, 2 out]
          }
          frame "Origin/Home" {
            n387 = Initialize Array(0.0 ("element"), w867) -> (w866:dbl[])
            n388 = Bundle By Name(cluster=w870, "Position target"=w866) -> (w869:T6)
          }
          frame Default {
            n389 = Unbundle By Name(w878) -> ("State"=w876:T5)
            n390 = Format Into String(format string="\nUnsupported command:%d,\nDefault frame", w876) -> (resulting string=w877:string)  [unwired: 2 in, 1 out]
            n391 = One Button Dialog(message=w877) -> ()  [unwired: 1 in, 1 out]
          }
        }
        n392 = call <vilib>:"General Error Handler.vi"("type of dialog (OK msg:1)"=w593, "error in (no error)"=w592, "[exception action] (none:0)"=w594, "[exception code]"=-1073807339) -> ("error out"=w599:errorcluster)  [unwired: 7 in, 4 out]
      }
      n393 = Merge Errors(w578, w573) -> (w574:errorcluster)
    }
  }
  "error out" <- w1
  n394 = while {
    tunnel: w4 -> [w1124]
    tunnel: w11 -> [w1127]
    tunnel: w5 -> [w1123]
    tunnel: w22 -> [w1125]
    tunnel: [w1123] -> w3
    i -> [w1122]
    stop <- w1128 stop-if-true
    # "Control queue"
    n395 = event shown="[6] \"X+\", \"X-\", \"Y+\", \"Y-\", \"Z+\", \"Z-\": Value Change" {
      selector: _ -> [_ _ _ _ _ _ _ _ _ _ _ _]
      dyn-events: _ -> [_ _ _ _ _ _ _ _ _ _ _ _]
      timeout: 50 -> [_ _ _ _ _ _ _ _ _ _ _ _]
      tunnel: [w1131 _ _ _ _ _ _ _ _ _ TRUE _] -> w1128
      tunnel: w1127 -> [w1144 _ _ _ _ _ _ _ _ _ _ _]
      tunnel: w1124 -> [w1143 w1163 w1174 w1184 w1188 w1199 w1226 w1232 w1234 w1240 w1243 w1246]
      tunnel: w1123 -> [w1136 _ _ _ _ _ _ _ _ _ _ _]
      tunnel: w1125 -> [w1135 w1162 w1173 _ _ _ w1225 _ _ _ _ _]
      tunnel: w1122 -> [_ _ _ _ _ _ _ _ _ w1236 _ _]
      event Timeout {
        # "Send return queue ref"
        n396 = event-data() -> ()  [unwired: 1 in, 1 out]
        n397 = Unbundle By Name(w1135) -> ("WaitStopReturn_Queue"=w1130:refnum<queue>)
        n398 = Not(x=w1144) -> (.not. x?=w1131:bool)
        n399 = Bundle By Name(cluster=T3 {"State"=enum."QueryStatus", "Params."=variant} ("element"), "Params."=w1136) -> (w1141:T3)
        n400 = Enqueue Element(queue=w1143, element=w1141) -> (error out=w1139:errorcluster)  [unwired: 2 in, 2 out]
        n401 = Dequeue Element(queue=w1136, timeout in ms (-1)=1000, error in (no error)=w1139) -> (element=w1137:T4, timed out?=w1138:bool)  [unwired: 2 out]
        n402 = case shown="False" w1138 {
          tunnel: w1137 -> [w1152 _]
          frame False {
            n403 = Unbundle By Name(w1152) -> ("Position"=→"Position":dbl[], "Velocity"=→"Velocity":dbl[], "Acceleration"=→"Acceleration":dbl[], "Moving"=→"Moving":bool)
          }
          frame True {
          }
        }
        n404 = Dequeue Element(queue=w1130, timeout in ms (-1)=0) -> (queue out=w1129:refnum<queue>, element=w1134:string, timed out?=w1133:bool)  [unwired: 1 in, 1 out]
        n405 = case "Non-blocking WaitStop in UI for testing" shown="False" w1133 {
          tunnel: w1134 -> [w1146 _]
          frame False {
            # "Non-blocking Wait for testing"
            n406 = Tick Count (ms)() -> (millisecond timer value=→"tick_stop":u32)
            "Returned_String" <- w1146
          }
          frame True {
          }
        }
        n407 = case "Release feedback queue if no UI" shown="True" w1131 {
          tunnel: w1129 -> [_ w1145]
          frame False {
          }
          frame True {
            n408 = Release Queue(queue=w1145) -> ()  [unwired: 2 in, 3 out]
          }
        }
      }
      event "Go": Value Change {
        n409 = Unbundle By Name(w1162) -> ("WaitStopReturn_Queue"=w1157:refnum<queue>, "SetPosition"=w1161:refnum<vi>)
        n410 = event-data() -> ()  [unwired: 1 in, 1 out]
        n411 = flat-sequence {
          tunnel: w1163 -> [w1170]
          tunnel: w1160 -> [w1167]
          tunnel: [w1166] -> w1159
          tunnel: [w1165] -> w1158
          frame #0 {
            n412 = Tick Count (ms)() -> (millisecond timer value=→"tick_start":u32)
            n413 = Bundle By Name(cluster=T3 {"State"=enum."MoveAbs_all", "Params."=variant} ("element"), "Params."=w1167) -> (w1168:T3)
            n414 = Enqueue Element(queue=w1170, element=w1168) -> (queue out=w1166:refnum<queue>, error out=w1165:errorcluster)  [unwired: 2 in, 1 out]
          }
        }
        n415 = property class="Arr (strict)"(reference=w1161) -> ("Value"=w1160:dbl[])  [unwired: 1 in, 2 out]
        n416 = local write "Returned_String"("Done" ("Returned_String")) -> ()
        n417 = local write "tick_stop"(u32 0 ("tick_stop")) -> ()
        n418 = Bundle By Name(cluster=T3 {"State"=enum."WaitStop", "Params."=variant} ("element"), "Params."=w1157) -> (w1154:T3)
        n419 = Enqueue Element(queue=w1159, element=w1154, error in (no error)=w1158) -> ()  [unwired: 1 in, 3 out]
      }
      event "Go_MoveRel": Value Change {
        n420 = event-data() -> ()  [unwired: 1 in, 1 out]
        n421 = Unbundle By Name(w1173) -> ("SetPosition"=w1172:refnum<vi>)
        n422 = flat-sequence {
          tunnel: w1174 -> [w1180]
          tunnel: w1171 -> [w1177]
          tunnel: [w1176] -> _
          tunnel: [w1175] -> _
          frame #0 {
            n423 = Bundle By Name(cluster=T3 {"State"=enum."MoveRel_all", "Params."=variant} ("element"), "Params."=w1177) -> (w1178:T3)
            n424 = Enqueue Element(queue=w1180, element=w1178) -> (queue out=w1176:refnum<queue>, error out=w1175:errorcluster)  [unwired: 2 in, 1 out]
          }
        }
        n425 = property class="Arr (strict)"(reference=w1172) -> ("Value"=w1171:dbl[])  [unwired: 1 in, 2 out]
      }
      event "SetPosition": Value Change {
        n426 = event-data() -> ("NewVal"=w1181:dbl[])  [unwired: 1 in]
        n427 = Bundle By Name(cluster=T3 {"State"=enum."MoveAbs_all", "Params."=variant} ("element"), "Params."=w1181) -> (w1182:T3)
        n428 = Enqueue Element(queue=w1184, element=w1182) -> ()  [unwired: 2 in, 3 out]
      }
      event "SetVelocity": Value Change {
        n429 = event-data() -> ("NewVal"=w1187:dbl[])  [unwired: 1 in]
        n430 = for {
          tunnel: w1187 -> [w1190] mode=indexing
          shift-right: [w1189] -> w1186
          shift-left: w1188 -> [w1189]
          i -> [w1196]
          n431 = Increment(x=w1196) -> (x+1=w1194:i32)
          n432 = Bundle By Name(cluster=cluster{"Axis":i32, "Velocity":dbl} {"Axis"=0, "Velocity"=0.0}, "Velocity"=w1190, "Axis"=w1194) -> (w1191:cluster{"Axis":i32, "Velocity":dbl})
          n433 = Bundle By Name(cluster=T3 {"State"=enum."SetVelocity", "Params."=variant} ("element"), "Params."=w1191) -> (w1193:T3)
          n434 = Enqueue Element(queue=w1189, element=w1193) -> ()  [unwired: 2 in, 3 out]
        }
        n435 = Enqueue Element(queue=w1186, element=T3 {"State"=enum."GetVelocity", "Params."=variant}) -> ()  [unwired: 2 in, 3 out]
      }
      event "SetAcceleration": Value Change {
        n436 = event-data() -> ("NewVal"=w1200:dbl[])  [unwired: 1 in]
        n437 = for {
          tunnel: w1200 -> [w1202] mode=indexing
          shift-right: [w1201] -> w1197
          shift-left: w1199 -> [w1201]
          i -> [w1208]
          n438 = Increment(x=w1208) -> (x+1=w1206:i32)
          n439 = Bundle By Name(cluster=cluster{"Axis":i32, "Acceleration":dbl} {"Axis"=0, "Acceleration"=0.0}, "Acceleration"=w1202, "Axis"=w1206) -> (w1203:cluster{"Axis":i32, "Acceleration":dbl})
          n440 = Bundle By Name(cluster=T3 {"State"=enum."SetAcceleration", "Params."=variant} ("element"), "Params."=w1203) -> (w1205:T3)
          n441 = Enqueue Element(queue=w1201, element=w1205) -> ()  [unwired: 2 in, 3 out]
        }
        n442 = Enqueue Element(queue=w1197, element=T3 {"State"=enum."GetAcceleration", "Params."=variant}) -> ()  [unwired: 2 in, 3 out]
      }
      event "X+", "X-", "Y+", "Y-", "Z+", "Z-": Value Change {
        n443 = event-data() -> ()  [unwired: 1 in, 1 out]
        n444 = Unbundle By Name(w1225) -> ("StepWidth"=w1224:refnum<vi>)
        n445 = property class="Ring (strict)"(reference=w1224) -> ("Value"=w1216:T10)  [unwired: 1 in, 2 out]
        n446 = Build Array("X+", "X-", "Y+", "Y-", "Z+", "Z-") -> (w1223:bool[])
        n447 = Search 1D Array(1D array=w1223, element=TRUE) -> (index of element=w1220:i32)  [unwired: 1 in]
        n448 = Index Array(array=dbl[] [1.0, -1.0, 1.0, -1.0, 1.0, -1.0], index=w1220) -> (element=w1219:dbl)
        n449 = Index Array(array=i32[] [1, 1, 2, 2, 3, 3], index=w1220) -> (element=w1215:i32)
        n450 = Multiply(x=w1216, y=w1219) -> (x*y=w1217:T10)
        n451 = Bundle By Name(cluster=cluster{"Axis":i32, "Position":dbl} {"Axis"=0, "Position"=0.0}, "Position"=w1217, "Axis"=w1215) -> (w1227:cluster{"Axis":i32, "Position":dbl})
        n452 = Bundle By Name(cluster=T3 {"State"=enum."MoveRel", "Params."=variant} ("element"), "Params."=w1227) -> (w1229:T3)
        n453 = Enqueue Element(queue=w1226, element=w1229) -> ()  [unwired: 2 in, 3 out]
      }
      event "STOP": Value Change {
        n454 = event-data() -> ()  [unwired: 1 in, 1 out]
        n455 = Enqueue Element(queue=w1232, element=T3 {"State"=enum."STOP", "Params."=variant}) -> ()  [unwired: 2 in, 3 out]
      }
      event "Home": Value Change {
        n456 = event-data() -> ()  [unwired: 1 in, 1 out]
        n457 = Enqueue Element(queue=w1234, element=T3 {"State"=enum."Origin/Home", "Params."=variant}) -> ()  [unwired: 2 in, 3 out]
      }
      event "MotorDisabled": Value Change {
        n458 = event-data() -> ()  [unwired: 1 in, 1 out]
        n459 = Not(x="MotorDisabled") -> (.not. x?=w1235:bool)
        n460 = Bundle By Name(cluster=T3 {"State"=enum."MotorEnable(1)", "Params."=variant} ("element"), "Params."=w1235) -> (w1238:T3)
        n461 = Enqueue Element(queue=w1240, element=w1238) -> ()  [unwired: 2 in, 3 out]
        "Numeric" <- w1236
      }
      event "Quit": Value Change {
        n462 = event-data() -> ()  [unwired: 1 in, 1 out]
        n463 = disable-structure shown="Disabled" {
          frame Disabled {
            n464 = property on="Quit" class="Bool (strict)"("Value"=FALSE ("Quit")) -> ()  [unwired: 2 in, 2 out]
          }
          frame Enabled {
          }
        }
        n465 = Enqueue Element(queue=w1243, element=T3 {"State"=enum."Quit", "Params."=variant}) -> ()  [unwired: 2 in, 3 out]
      }
      event "ClearErr": Value Change {
        n466 = event-data() -> ()  [unwired: 1 in, 1 out]
        n467 = Enqueue Element(queue=w1246, element=T3 {"State"=enum."ClearErr", "Params."=variant}) -> ()  [unwired: 2 in, 3 out]
      }
    }
  }
  n468 = Release Queue(queue=w2, error in (no error)=w1) -> ()  [unwired: 1 in, 3 out]
  n469 = Release Queue(queue=w3, error in (no error)=w1) -> ()  [unwired: 1 in, 3 out]
